vi "TLB Native Dynamic Events ver 0.15a.vi"() -> ()   [LabVIEW 2018]
uses:
  Labview Training Phase 2/Enum Controls/States for Action Engine.ctl
  TLB Type Definitions/State Type Definitions, for 0.26g versions and later 2.ctl
  TLB Type Definitions/Intruction Type Definitions.ctl
  TLB Type Definitions/Encoder cluster.ctl
  TLB Type Definitions/PING CLUSTER.ctl
  <vilib>/Studica/Studica Toolkit/NavX/NavX.lvlib
  <vilib>/Studica/Studica Toolkit/Background/DIO Channel.ctl
  Underlying VI's/NavX VI/navX type def.ctl
  <vilib>/myRIO/Instrument Drivers/Utilities/Utilities.lvlib
  <vilib>/Studica/Studica Toolkit/Background/I2C Channel.ctl
  TLB Type Definitions/Vision cluster.ctl
  <vilib>/NI_Real-Time Target Support.lvlib
  TLB Type Definitions/Stepper cluster.ctl
  Experimental VI's/Archived VI's/MOTOR CONTROL NO PID Type Def.ctl
  Underlying VI's/I2C Master VI/I2C MASTER Type Def.ctl
  Underlying VI's/I2C Master VI/I2C_MASTER_WRITE_NEW Type Def.ctl
  <vilib>/userdefined/High Color/IMAQdx.ctl
  Underlying VI's/I2C Master VI/Arduino_Interfacing.ctl
  TLB Type Definitions/Yaw Cluster.ctl
  Experimental VI's/Archived VI's/MOTOR CONTROL NO PID AE DATA ENTRY MODE Type def.ctl
  Experimental VI's/Archived VI's/MOTOR CONTROL NO PID AE DIRECTIONS type def.ctl
  Underlying VI's/Elasped Timer/Control.ctl
  TLB Type Definitions/Time cluster.ctl
  TLB Type Definitions/Y Stepper cluster.ctl
  Underlying VI's/Modified webcam FGV/Webcam AE.ctl
  <vilib>/Utility/RT CPU Load.ctl
panel:
  out "Does it leave this state?":bool
  out "Is object in range to pick up?":bool
  out "Does this get triged":bool
  out "Stepper position reached?":bool
  out "Cluster":T1
  out "Object Center Coordinates":cluster{"x":sgl, "y":sgl}
  out "Object detection cluster":T2
  out "Time up flag":bool
  out "Speed & distance":T3
  out "Task selection":u8
  in  "Object recognition mode":enum16{"Ball", "Soap", "Gel", "Pipe", "None"}(ring)
  out "NavX Readings":T4
  out "Arduino Data":T5
  out "CPU loads":T6[](array[typedef]) {"ISR (%)" format="%#.2f"; "Idle (%)" format="%#.2f"; "Background (%)" format="%#.2f"; "Normal (%)" format="%#.2f"; "Above Normal (%)" format="%#.2f"; "High (%)" format="%#.2g"; "Timed Structures (%)" format="%#.2g"; "Time Critical (%)" format="%#.2g"; "Total (%)" format="%#.2g"}
  out "TASK ENABLE":bool
  out "Rising Edge":bool
  in  "Green LED":bool
  out "Obstacle detected":bool
  out "I2C Error":errorcluster
  out "State Logic":T7=enum."Startup"
  out "elements":T8[](array[typedef])
  in  "STOP TASK":bool
  in  "OK Button":bool
  in  "STOP":bool
  out "error out":errorcluster
  out "Action Queue Items":i32
  out "State Logic Queue Items":i32
  out "Action Queues items":string[](array[string])=["Hardware reset", "Software reset", ""]
  out "Action State":string
  # "VISION"
  # "System Health Status Update"
  # "TLB FRAMEWORK STATUS"
  # "Test Programme written by Calvin Loke    Dated: 28 Aug 2019\nTest Programme revised by Dr Alex See   Dated 30 Aug 2019\n\nRevision date: 20/03/2020\nProgramme version:   TLB Native Dynamic Events ver 0.15a"
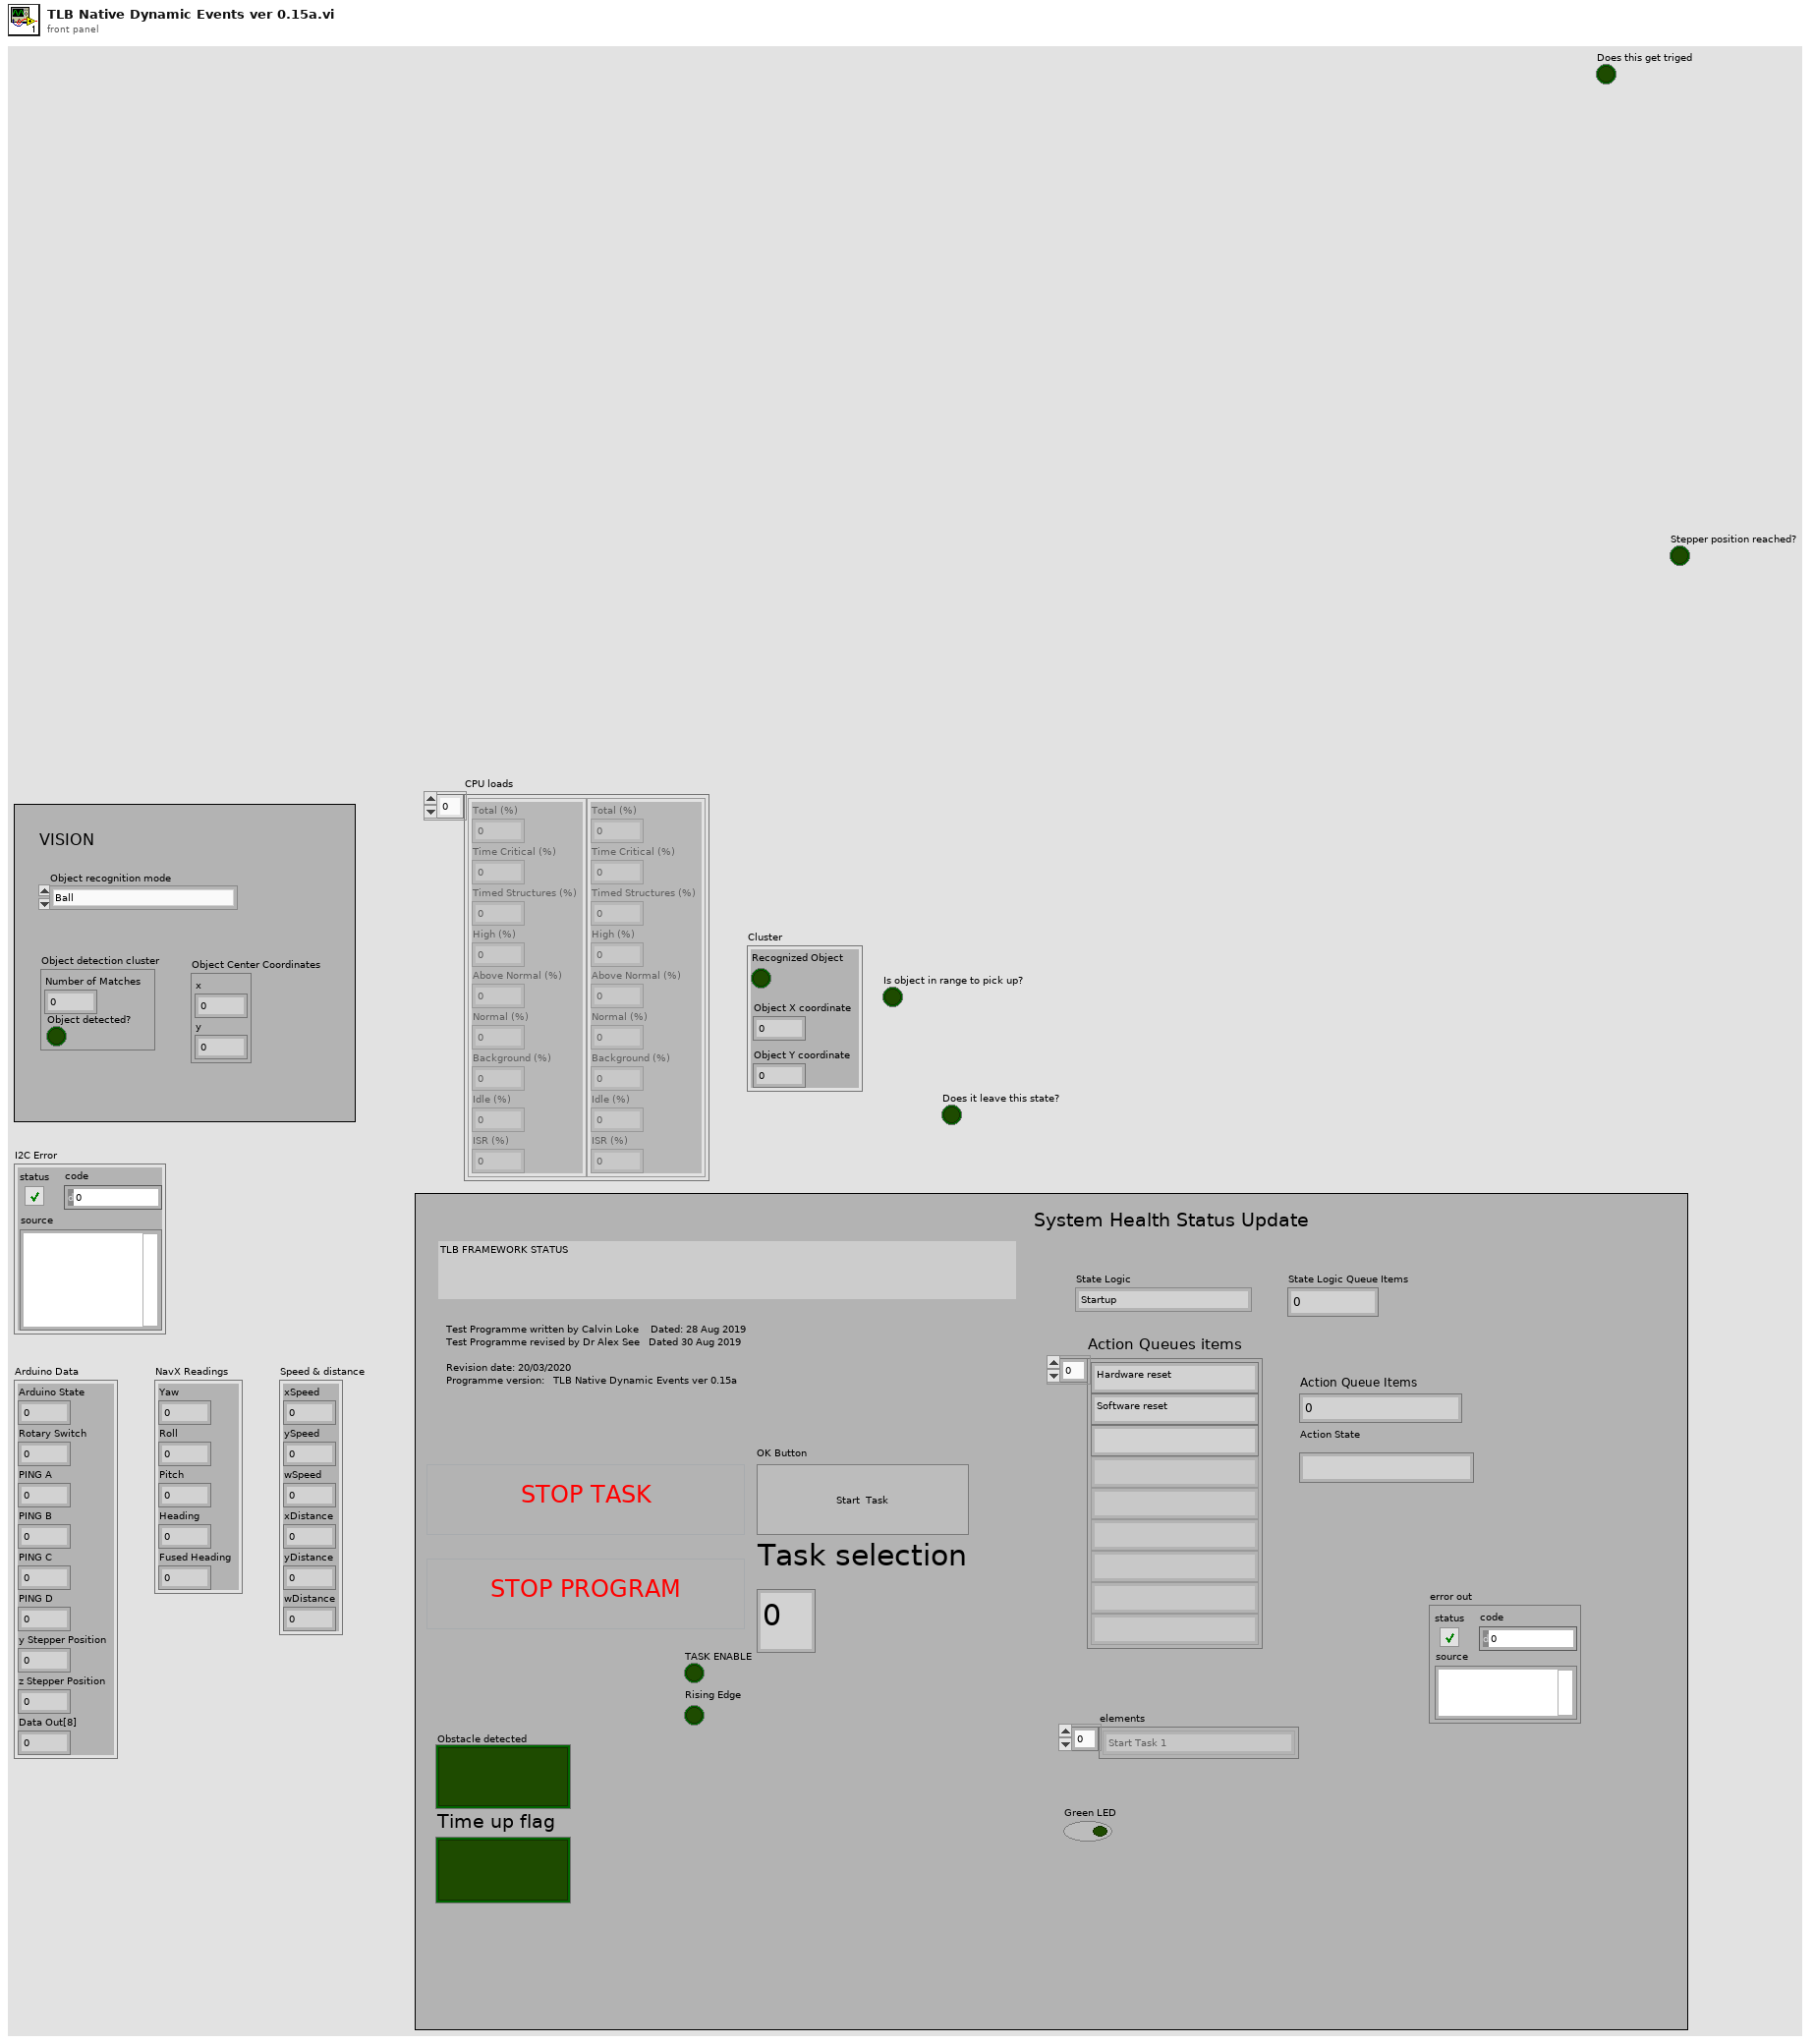
[diagram p1: front panel]
types:
  T1 = typedef "Vision cluster.ctl" = cluster{"Recognized Object":bool, "Object X coordinate":dbl, "Object Y coordinate":dbl}
  T2 = cluster{"Number of Matches":i32, "Object detected?":bool}
  T3 = cluster{"xSpeed":dbl, "ySpeed":dbl, "wSpeed":dbl, "xDistance":dbl, "yDistance":dbl, "wDistance":dbl}
  T4 = cluster{"Yaw":dbl, "Roll":dbl, "Pitch":dbl, "Heading":dbl, "Fused Heading":dbl}
  T5 = cluster{"Arduino State":u8, "Rotary Switch":u8, "PING A":u8, "PING B":u8, "PING C":u8, "PING D":u8, "y Stepper Position":u8, "z Stepper Position":u8, "Data Out[8]":u8}
  T6 = typedef "NI_Real-Time Target Support.lvlib/RT CPU Load.ctl" = cluster{"Total (%)":dbl, "Time Critical (%)":dbl, "Timed Structures (%)":dbl, "High (%)":dbl, "Above Normal (%)":dbl, "Normal (%)":dbl, "Background (%)":dbl, "Idle (%)":dbl, "ISR (%)":dbl}
  T7 = typedef "State Type Definitions, for 0.26g versions and later 2.ctl" = enum16{"None", "Startup", "Move to Angle", "True Stop", "Idle", "Shutdown", "Task 1A", "Task 1B", "Task 2:Raise Arm", "Task 2:Sensor Mode", "Task 2:Reverse Mode", "Task 3", "Task 4_A", "Task 4_B", "Task 4_C", "Task 4_D", "Task 5A", "Task 5B", "Task 5C", "Task 5D", "Task 5E: POSITION ARM", "Task 5F: ARM GRAB HEIGHT", "Task 5G: CLOSE CLAW", "Task 5H: RAISE ARM", "Task 6_A", "Task 6_B", "Task 7", "Task 8A: RAISE ARM", "Task 8B: MOVE TO BOX", "Task 8C: CAM BURST", "Task 8D: PROCESS IMAGE", "Task 8E: ROBOT ADJUST", "Task 8F: CAM BURST 2", "Task 8G: PROCESS IMAGE 2", "Task 8H: ARM ADJUST", "Task 8I: ARM GRAB HEIGHT", "Task 8J: CLOSE CLAW", "Task 8K: RAISE MY SWORD", "Task 9A: Raise Arm", "Task 9B: Rotate to Angle", "Task 9C: Detect Box", "Task 9D: MOVE FORWARD", "Task 9E: MOVE LEFT", "Task 9F: SCAN BOX", "Task 9G: MOVE RIGHT", "Task 9H: SCAN BOX 2", "Task 9I: ROTATE 90 CW", "Task 9J: FORWARD", "Task 9K: RAM WALL", "Task 9L: MOVE RIGHT", "Task 9M: SCAN BOX 3", "Task 9M: MOVE RIGHT", "Task 9N: SCAN BOX 4", "PENIS", "PENIS 2", "PENIS 3", "Task 9R: PROCESS COLOUR", "Task A1: Task 9 Open cam", "Task A2: Task 9 Move Arm", "Task A3: Task 9 Set Timer", "Task A4: Tasl 9 Capture images", "Task A5: Task 9 Close camera", "Task A6: Process Colour", "Task A7: Dispose Camera Buffer"}
  T8 = typedef "Intruction Type Definitions.ctl" = enum16{"None", "Start Task 1", "Start Task 2", "Start Task 3", "Start Task 4", "Start Task 5", "Start Task 6", "Start Task 7", "Start Task 8 - BALL", "Start Task 8 - Gel", "Start Task 8 - Pipe", "Start Task 8 - Soap", "Start Task 9", "Start Task A", "Start Task B", "Exit"}
  T9 = typedef "Y Stepper cluster.ctl" = cluster{"yStepper desired":u8}
  T10 = typedef "Time cluster.ctl" = cluster{"Time up flag":bool, "SET TIME TO CHECK":dbl}
  T11 = typedef "Yaw Cluster.ctl" = cluster{"Yaw":dbl, "Compass":dbl}
  T12 = typedef "Stepper cluster.ctl" = cluster{"y Stepper Position":u8, "z Stepper Position":u8}
  T13 = typedef "DIO Channel.ctl" = enum16{"Not Connected", "A/DIO1", "A/DIO2", "A/DIO3", "A/DIO4", "A/DIO5", "A/DIO6", "A/DIO7", "A/DIO13", "B/DIO1", "B/DIO2", "B/DIO3", "B/DIO4", "B/DIO5", "B/DIO6", "B/DIO7", "B/DIO13", "C/DIO0", "C/DIO1", "C/DIO2", "C/DIO3", "C/DIO4", "C/DIO5", "C/DIO6", "C/DIO7"}
  T14 = typedef "PING CLUSTER.ctl" = cluster{"PING_A":u8, "PING_B":u8, "PING_C":u8, "PING_D":u8}
  T15 = typedef "Encoder cluster.ctl" = cluster{"xDistance":dbl, "yDistance":dbl, "wDistance":dbl}
  T16 = cluster{"DIO Channel":T13, "FPGA VI Reference Out":refnum<k20>}
  T17 = typedef "MOTOR CONTROL NO PID AE DATA ENTRY MODE Type def.ctl" = enum16{"Initialize", "Reset Encoders", "Write to motors", "Read from Encoders"}
  T18 = typedef "navX type def.ctl" = enum16{"Get i2C reference", "Read Values", "Zero Yaw"}
  T19 = typedef "Arduino_Interfacing.ctl" = enum16{"Initialize", "Write to Arduino", "Read From Arduino"}
  T20 = typedef "I2C Channel.ctl" = enum16{"Not Connected", "A", "B"}
  T21 = typedef "States for Action Engine.ctl" = enum16{"Initialize", "Write", "Read"}
  T22 = cluster{"I2C Ref Out":cluster{"I2C Channel":T20, "FPGA VI Reference Out":refnum<k20>}, "Connected":bool, "Slave Address (7-bit)":u8, "Registry":u8[]}
  T23 = typedef "IMAQ Image.ctl" = refnum<image>
  T24 = typedef "State Type Definitions.ctl" = enum16{"None", "Startup", "Move to Angle", "True Stop", "Idle", "Shutdown", "Task 1", "Task 2", "Task 3", "Task 4_A", "Task 4_B", "Task 4_C", "Task 4_D", "Task 5_A", "Task 5 _B", "Task 5_C", "Task 5_D", "Task 5_D_Error", "Task 5D_Error_Right", "Task 5D_Error_Left", "Task 5_E", "Task 5_F", "Task 5F_Error", "Task 5G", "Task 5H", "Task 5I", "Task 6_A", "Task 6_B", "Task 7", "Task 8", "Task 9", "Task A", "Task B"}
  T25 = typedef "MOTOR CONTROL NO PID AE DIRECTIONS type def.ctl" = enum16{"y-axis movement", "x-axis movement", "Rotate", "Stop"}
  T26 = typedef "Control.ctl" = enum16{"Start", "Pause", "Initialize"}
  T27 = typedef "I2C_MASTER_WRITE_NEW Type Def.ctl" = enum16{"Ultrasonic sensors", "Stepper origin", "zStepper 13.3k", "zStepper 13k", "zStepper 12k", "zStepper 11k", "zStepper 10k", "zStepper 9k", "zStepper 8k", "zStepper 7k", "zStepper 6k", "zStepper 5k", "zStepper 4k", "zStepper 3k", "zStepper 2k", "zStepper 1k", "zStepper 900", "zStepper 800", "zStepper 700", "zStepper 600", "zStepper 500", "zStepper 400", "zStepper 300", "zStepper 200", "zStepper 100", "zStepper 0", "yStepper control", "Open Claw", "Close Claw", "Soft Reset"}
  T28 = typedef "Webcam AE.ctl" = enum16{"Initialize Camera", "Open Camera", "Continuous Acquisition", "Close Camera", "Retrieve Image", "Dispose Camera Image Buffer"}
  T29 = typedef "IMAQdx.ctl" = refnum<k21>
  T30 = typedef "Webcam AE.ctl" = enum16{"Initialize Camera", "Open Camera", "Continuous Acquisition", "Close Camera", "Retrieve Image", "Dispose Image Buffers"}
  T31 = typedef "MOTOR CONTROL NO PID Type Def.ctl" = enum16{"Init", "Front Back", "Left Right", "Rotate", "Stop", "Latch"}
  T32 = typedef "I2C MASTER Type Def.ctl" = enum16{"Last State", "Mode 0", "Mode 1", "Mode 2", "Mode 3", "Mode 4", "Mode 5", "Mode 6", "Mode 7", "Mode 8", "Mode 9", "Mode 10"}
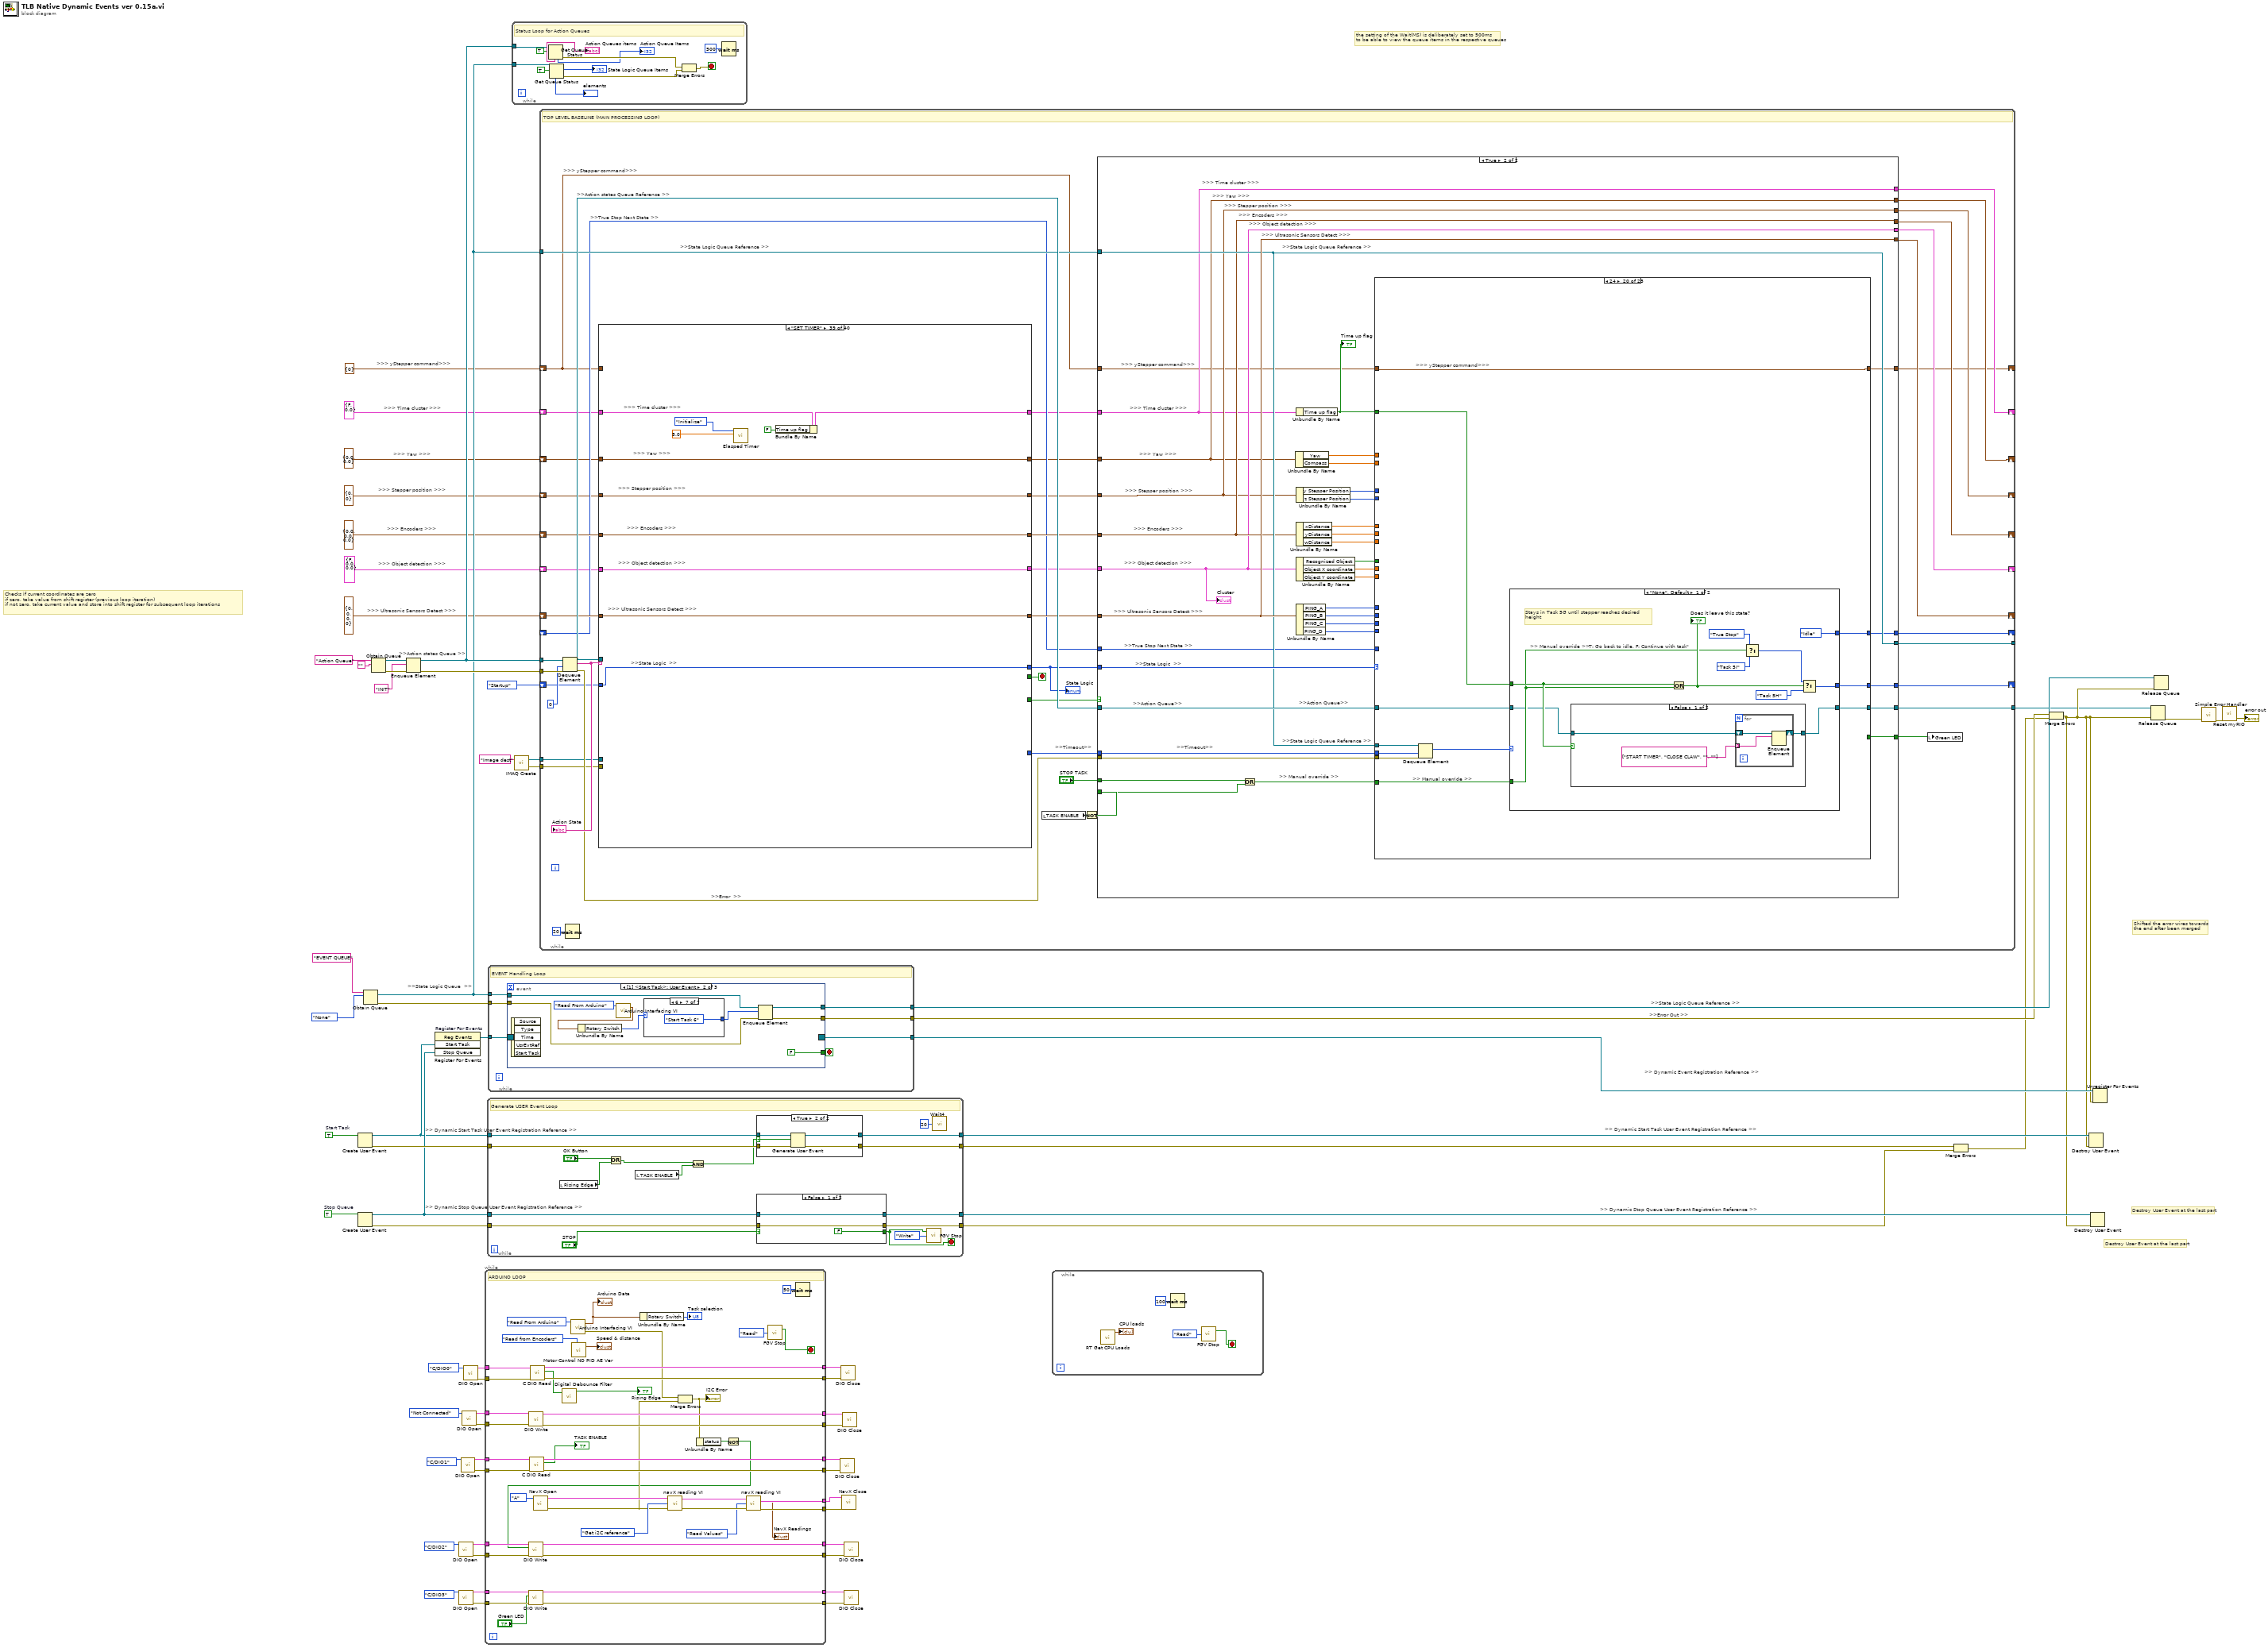
[diagram p0: block diagram]
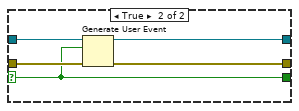
[diagram p2: hidden frame]
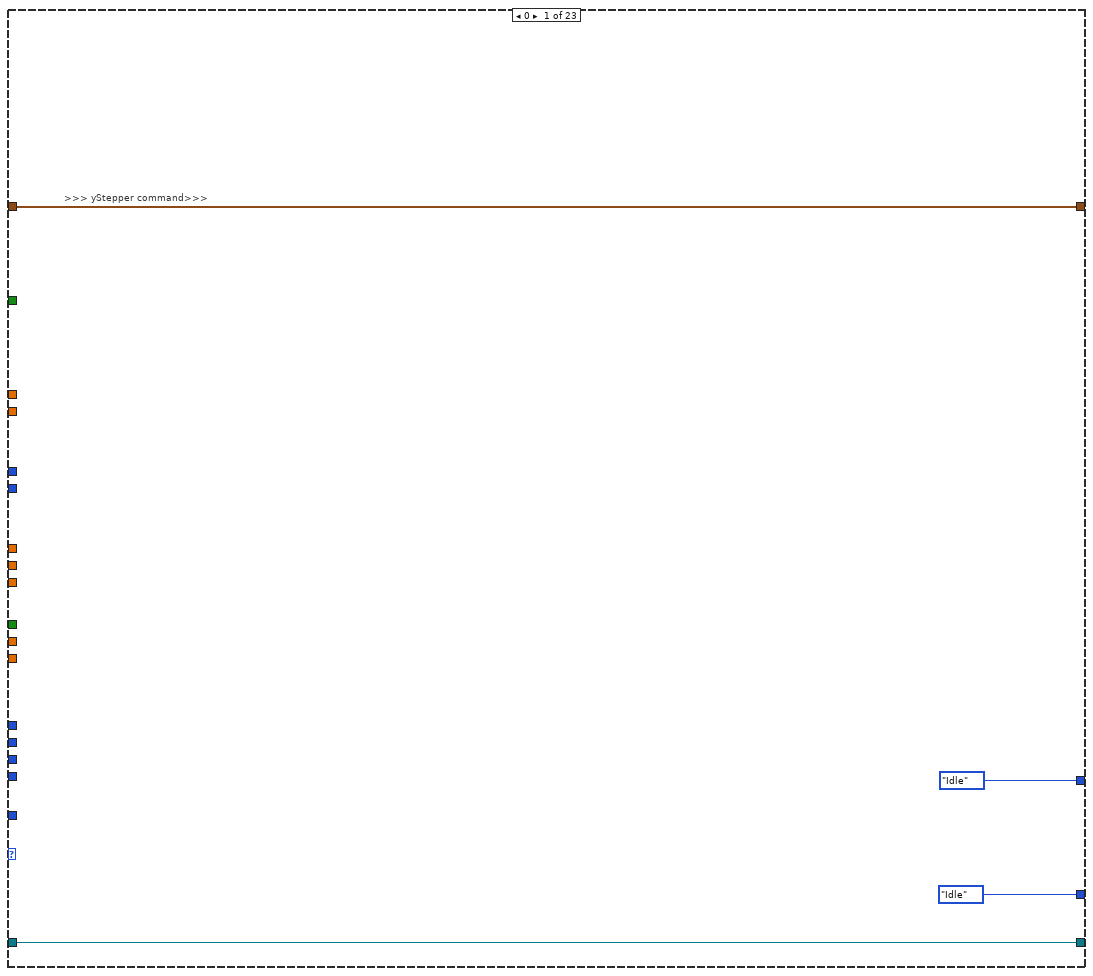
[diagram p5: hidden frame]
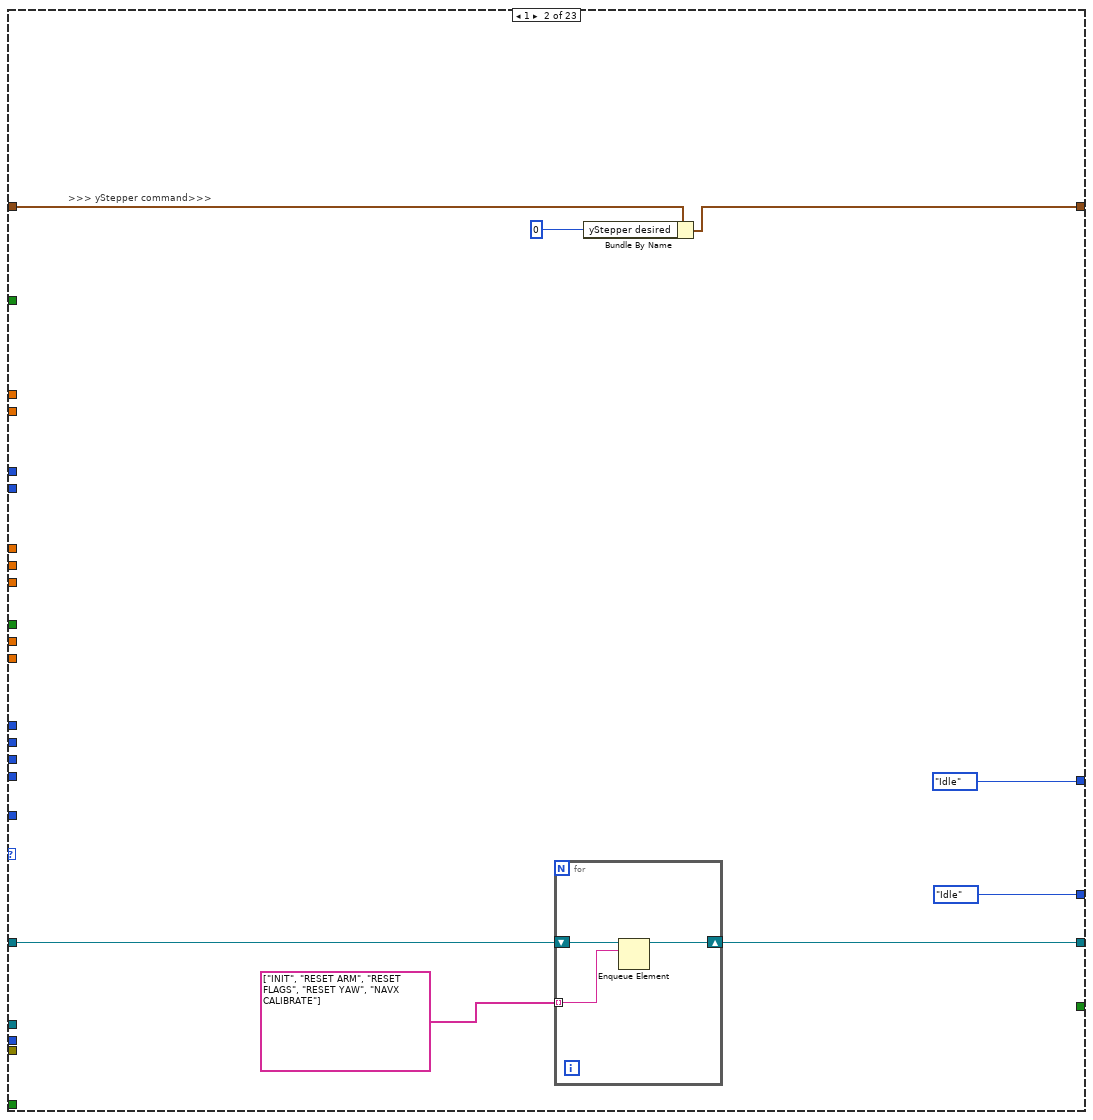
[diagram p6: hidden frame]
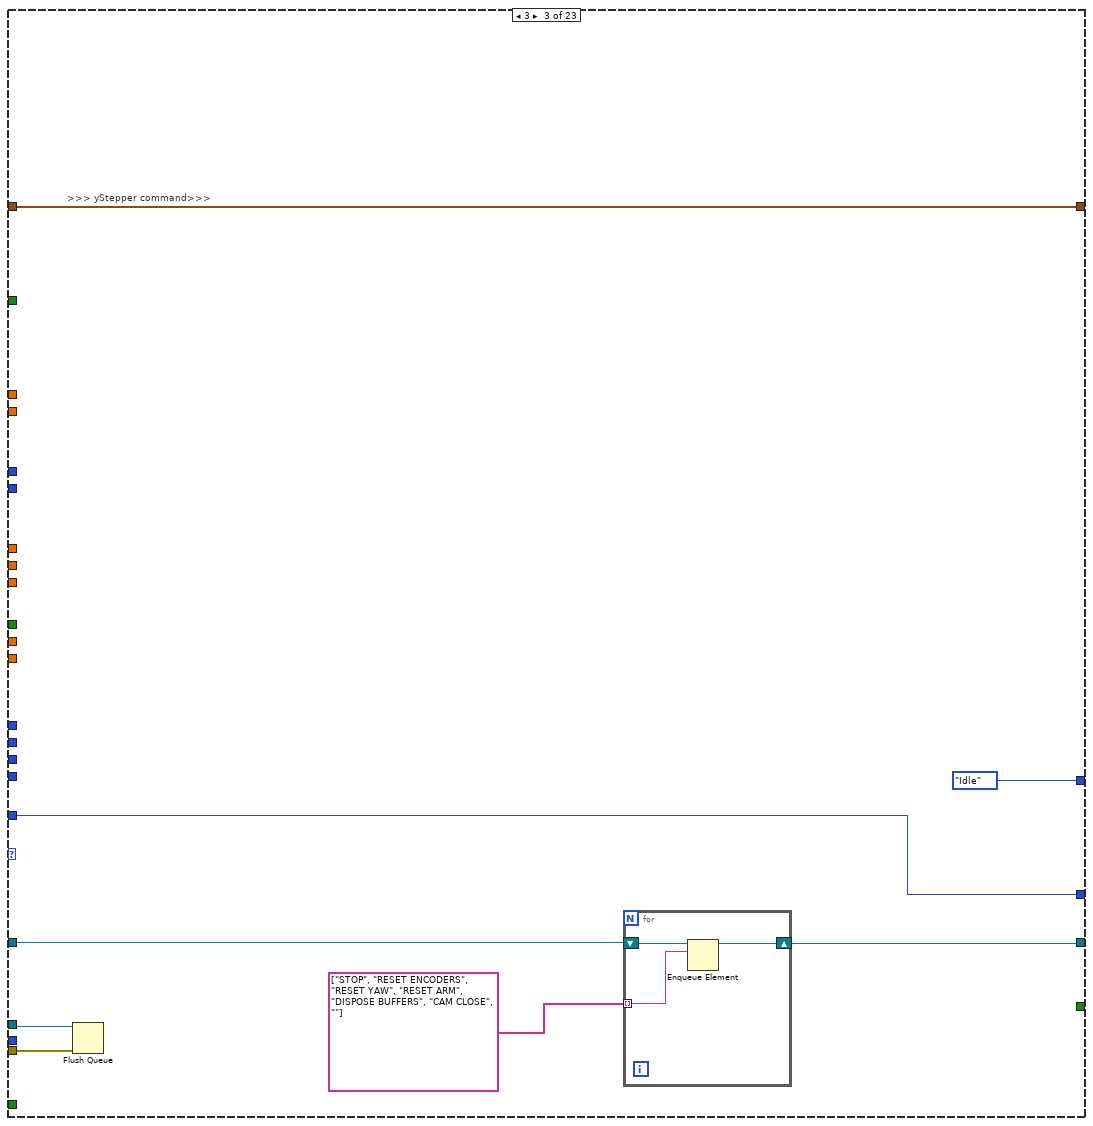
[diagram p7: hidden frame]
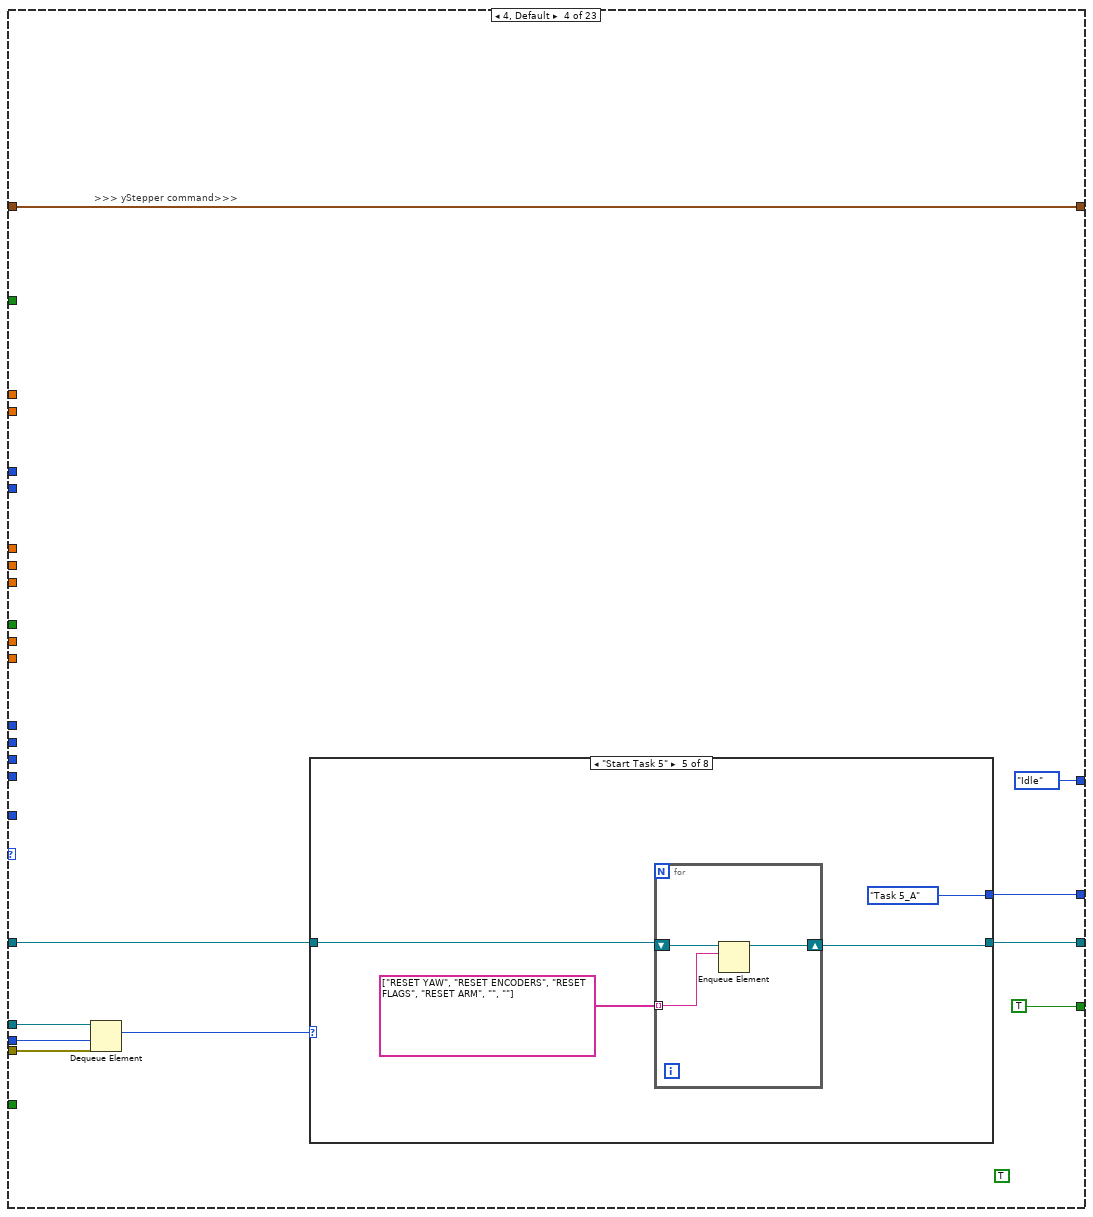
[diagram p8: hidden frame]
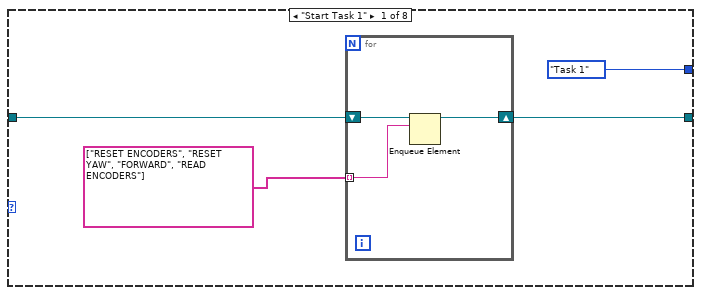
[diagram p9: hidden frame]
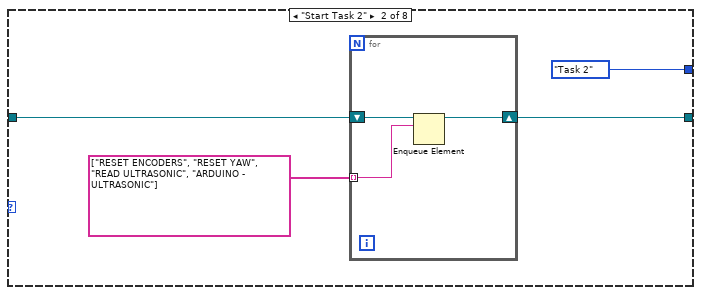
[diagram p10: hidden frame]
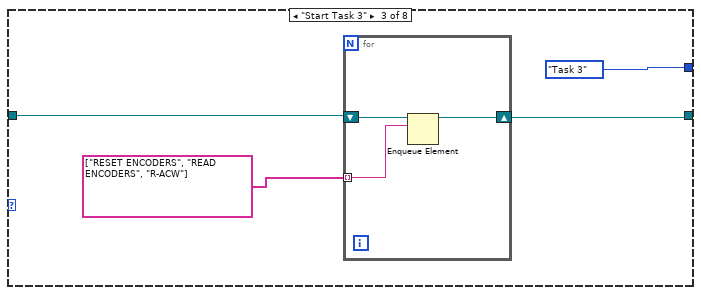
[diagram p11: hidden frame]
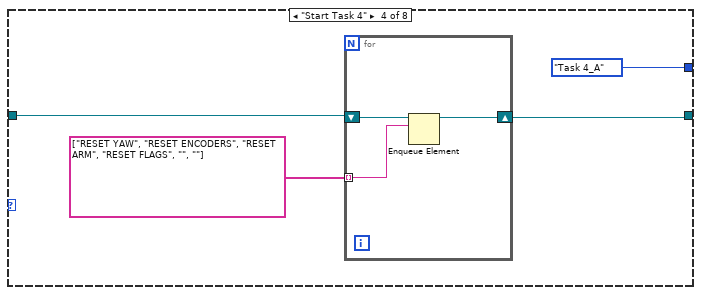
[diagram p12: hidden frame]
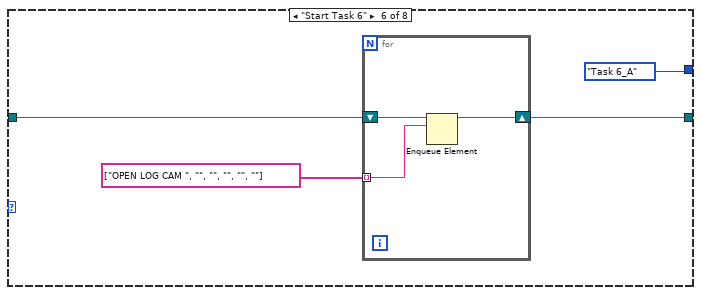
[diagram p13: hidden frame]
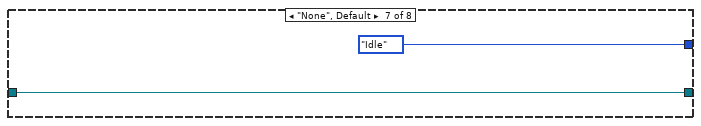
[diagram p14: hidden frame]
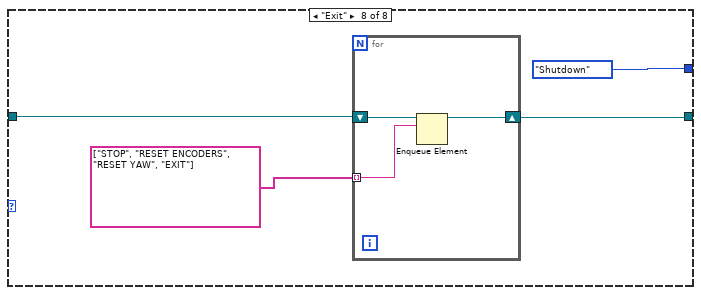
[diagram p15: hidden frame]
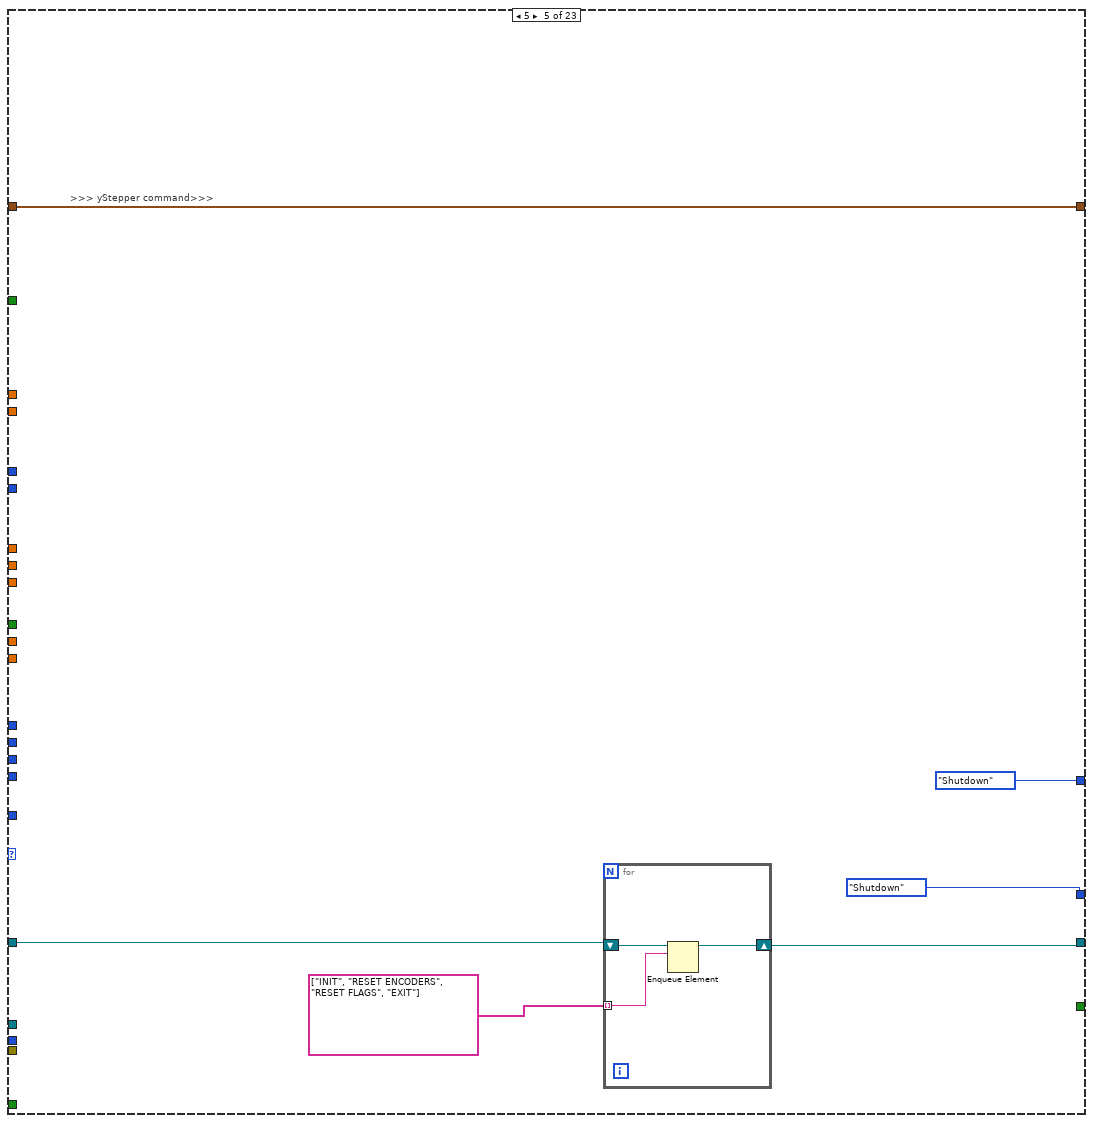
[diagram p16: hidden frame]
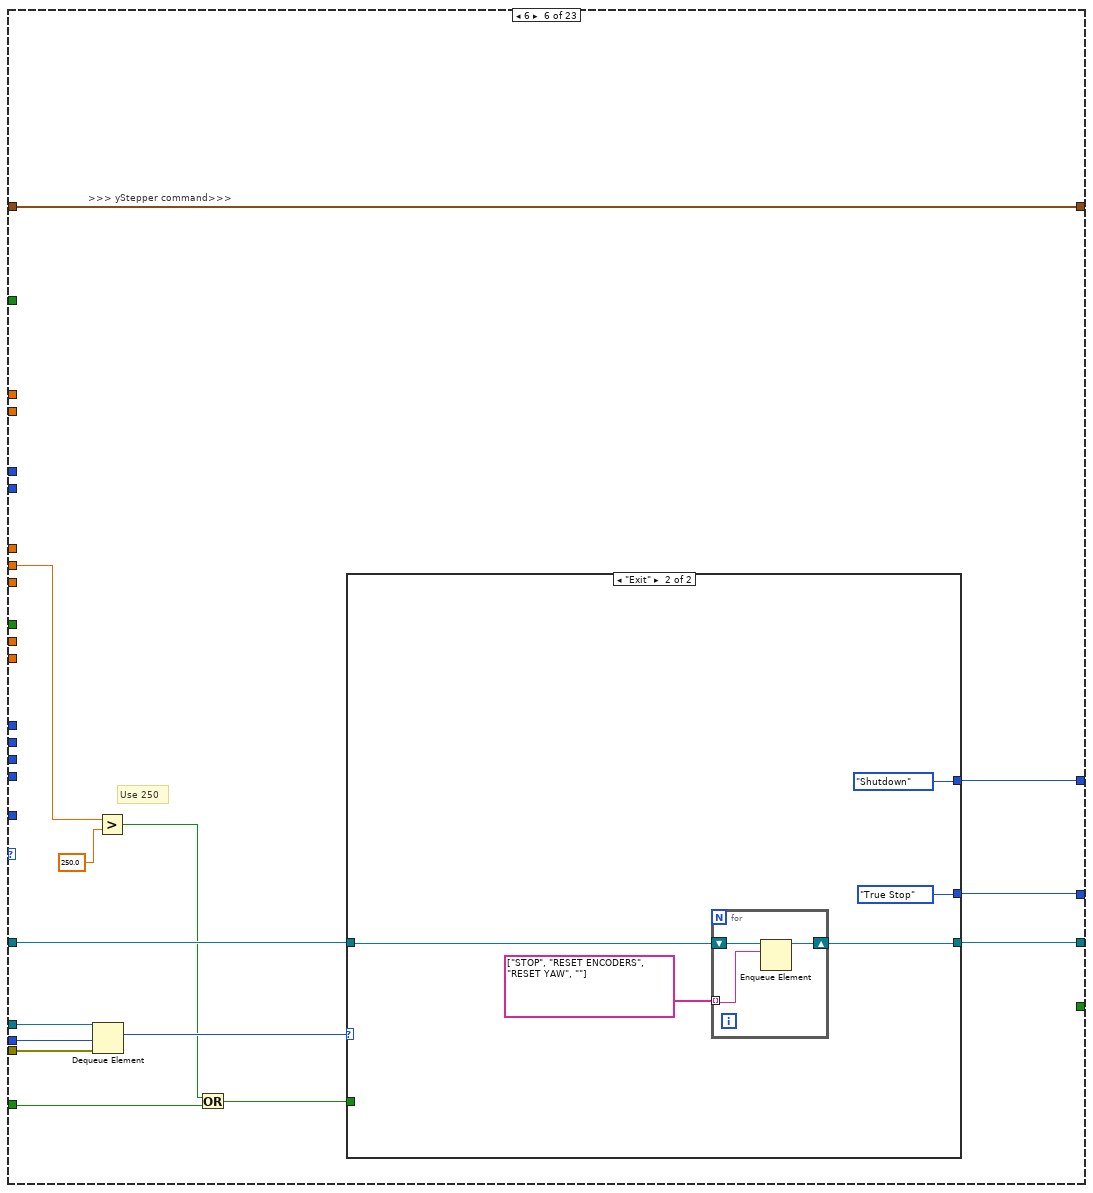
[diagram p17: hidden frame]
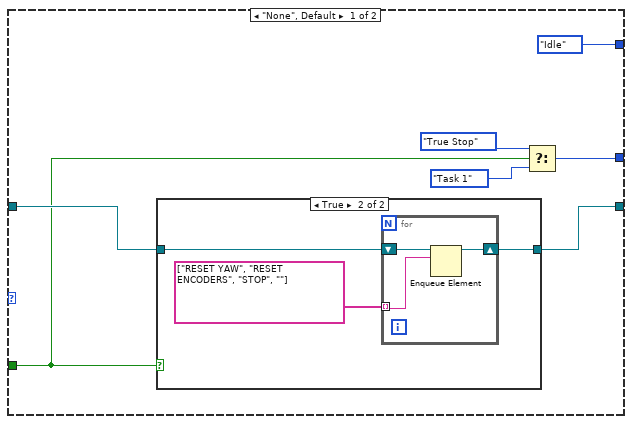
[diagram p18: hidden frame]
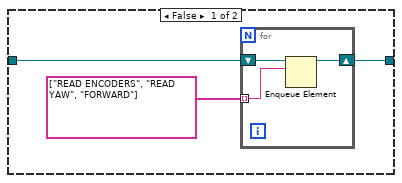
[diagram p19: hidden frame]
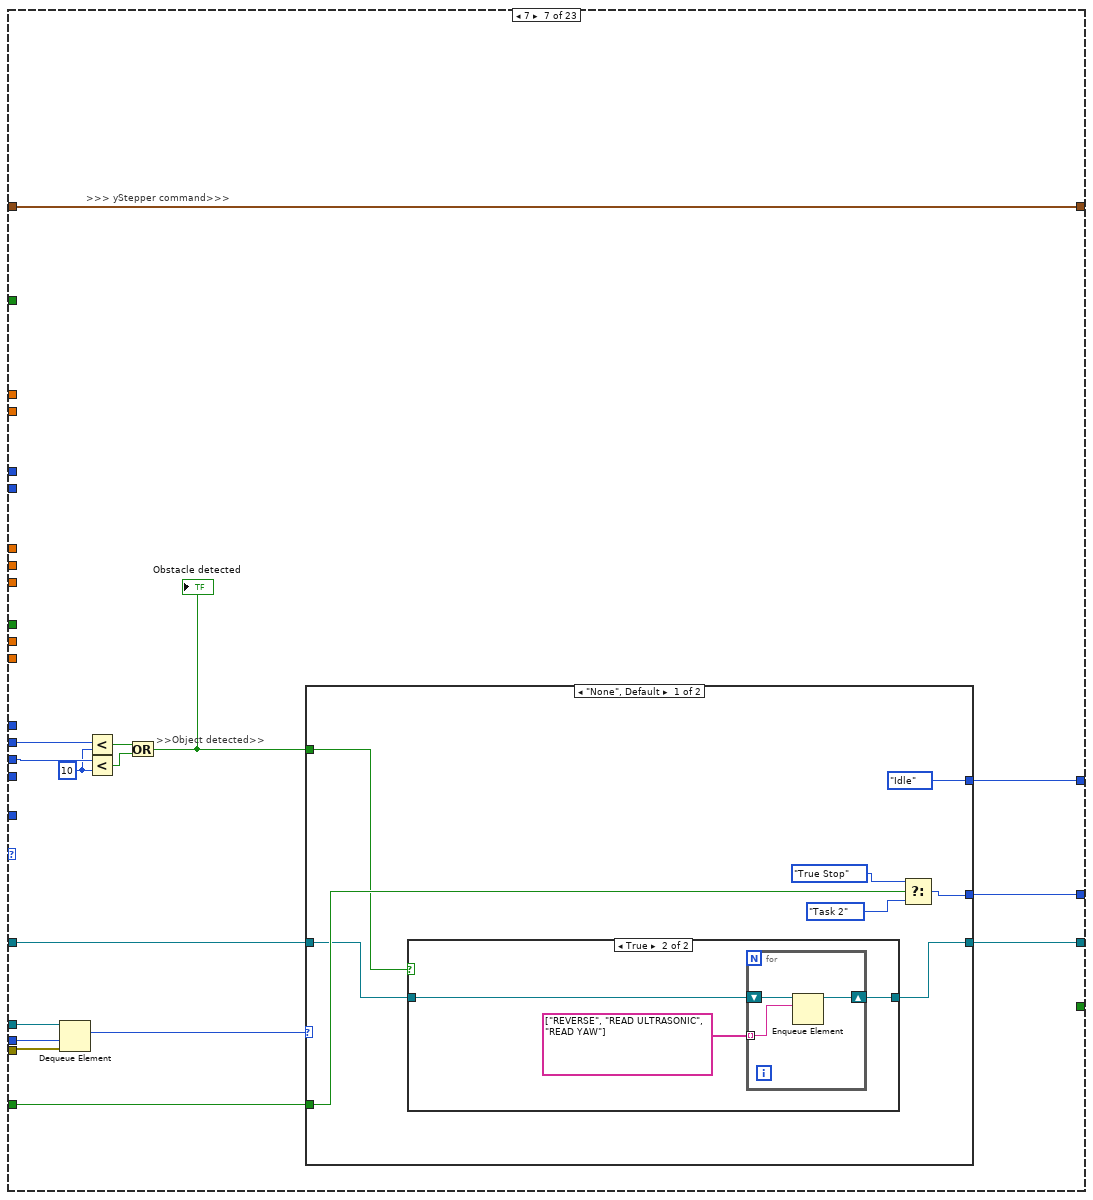
[diagram p20: hidden frame]
diagram:
  w69 = TRUE  # Stop Queue
  w68 = TRUE  # Start Task
  # "Checks if current coordinates are zero\nif zero, take value from shift register (previous loop iteration)\nif not zero, take current value and store into shift register for subsequent loop iterations"
  # ">>> yStepper command>>>"
  # ">>> Time cluster >>>"
  # ">>> Yaw >>>"
  # ">>> Stepper position >>>"
  # ">>> Encoders >>>"
  # ">>> Object detection >>>"
  # ">>> Ultrasonic Sensors Detect >>>"
  # "the setting of the Wait(MS) is deliberately set to 500ms\nto be able to view the queue items in the respective queues"
  # ">>Error Out >>"
  # ">> Dynamic Stop Queue User Event Registration Reference >>"
  # ">> Dynamic Start Task User Event Registration Reference >>"
  # ">> Dynamic Stop Queue User Event Registration Reference >>"
  # ">> Dynamic Start Task User Event Registration Reference >>"
  # ">> Dynamic Event Registration Reference >>"
  # ">>Action states Queue >>"
  # ">>State Logic Queue  >>"
  # ">>State Logic Queue Reference >>"
  # "Destroy User Event at the last part"
  # "Destroy User Event at the last part"
  # "Shifted the error wires towards\nthe end after been merged"
  n1 = Create User Event(user event datatype=w68) -> (user event=w60:refnum<user-event>, error out=w65:errorcluster)  [unwired: 1 in]
  n2 = Create User Event(user event datatype=w69) -> (user event=w61:refnum<user-event>, error out=w64:errorcluster)  [unwired: 1 in]
  n3 = Obtain Queue(name (unnamed)="EVENT QUEUE", element data type=Intruction_Type_Definitions."None" ("Enum")) -> (queue out=w46:refnum<queue>, error out=w52:errorcluster)  [unwired: 3 in, 1 out]
  n4 = Obtain Queue(name (unnamed)="Action Queue", element data type="") -> (queue out=w55:refnum<queue>, error out=w51:errorcluster)  [unwired: 3 in, 1 out]
  n5 = Enqueue Element(queue=w55, element="INIT", error in (no error)=w51) -> (queue out=w47:refnum<queue>, error out=w50:errorcluster)  [unwired: 1 in, 1 out]
  n6 = register-events "Register For Events"(w60, w61) -> (reference out=w59:refnum<event-registration>)  [unwired: 2 in, 1 out]
  n7 = call <vilib>:"DIO Open.vi"("DIO Channel"=DIO_Channel."C/DIO2") -> ("error out"=w14:errorcluster, "DIO Info Out"=w15:T16)  [unwired: 9 in]
  n8 = call <vilib>:"DIO Open.vi"("DIO Channel"=DIO_Channel."C/DIO3") -> ("error out"=w9:errorcluster, "DIO Info Out"=w10:T16)  [unwired: 9 in]
  n9 = call <vilib>:"DIO Open.vi"("DIO Channel"=DIO_Channel."C/DIO1") -> ("error out"=w25:errorcluster, "DIO Info Out"=w26:T16)  [unwired: 9 in]
  n10 = call <vilib>:"DIO Open.vi"("DIO Channel"=DIO_Channel."Not Connected") -> ("error out"=w30:errorcluster, "DIO Info Out"=w32:T16)  [unwired: 9 in]
  n11 = call <vilib>:"DIO Open.vi"("DIO Channel"=DIO_Channel."C/DIO0") -> ("error out"=w35:errorcluster, "DIO Info Out"=w38:T16)  [unwired: 9 in]
  n12 = while {
    tunnel: w38 -> [w112]
    tunnel: [w111] -> w36
    tunnel: w35 -> [w110]
    tunnel: [w109] -> w34
    tunnel: w32 -> [w106]
    tunnel: [w105] -> w31
    tunnel: w30 -> [w104]
    tunnel: [w103] -> w29
    tunnel: [w102] -> w27
    tunnel: w26 -> [w101]
    tunnel: w25 -> [w100]
    tunnel: [w99] -> w24
    tunnel: w15 -> [w93]
    tunnel: w14 -> [w92]
    tunnel: [w91] -> w13
    tunnel: [w90] -> w12
    tunnel: w10 -> [w89]
    tunnel: w9 -> [w88]
    tunnel: [w87] -> w8
    tunnel: [w86] -> w7
    tunnel: [w80] -> w4
    tunnel: [w79] -> w5
    stop <- w114 stop-if-true
    # "ARDUINO LOOP"
    n13 = call <vilib>:"DIO Write.vi"("error in (no error)"=w88, "Input"="Green LED", "DIO Info In"=w89) -> ("error out"=w86:errorcluster, "DIO Info Out"=w87:T16)  [unwired: 7 in]
    n14 = call <vilib>:"DIO Write.vi"("error in (no error)"=w104, "DIO Info In"=w106) -> ("error out"=w103:errorcluster, "DIO Info Out"=w105:T16)  [unwired: 8 in]
    n15 = call <vilib>:"C DIO Read.vi"("error in (no error)"=w100, "DIO Info In in"=w101) -> ("error out"=w99:errorcluster, "IN"=→"TASK ENABLE":bool, "DIO Info In out"=w102:T16)  [unwired: 7 in]
    n16 = call <vilib>:"C DIO Read.vi"("error in (no error)"=w110, "DIO Info In in"=w112) -> ("error out"=w109:errorcluster, "IN"=w108:bool, "DIO Info In out"=w111:T16)  [unwired: 7 in]
    n17 = call <vilib>:"NavX Open.vi"("I2C Channel"=I2C_Channel."A") -> ("error out"=w95:errorcluster, "NavX Info"=w97:T22)  [unwired: 9 in]
    n18 = call "Digital Debounce Filter.vi"("Boolean input"=w108) -> ("Rising Edge"=→"Rising Edge":bool)  [unwired: 1 in, 2 out]
    n19 = call "Arduino Interfacing VI.vi"("AE Mode"=Arduino_Interfacing."Read From Arduino") -> ("error out"=w83:errorcluster, "Arduino Data"=w76:T5)  [unwired: 3 in]
    "Arduino Data" <- w76
    n20 = call "Motor Control NO PID AE Ver.vi"("AE Mode"=MOTOR_CONTROL_NO_PID_AE_DATA_ENTRY_MODE_Type_def."Read from Encoders") -> ("Speed & distance"=→"Speed & distance":T3)  [unwired: 4 in, 1 out]
    n21 = Unbundle By Name(w76) -> ("Rotary Switch"=→"Task selection":u8)
    n22 = call "navX reading VI.vi"("NavX Info In"=w97, "Mode"=navX_type_def."Get i2C reference", "error in (no error)"=w95) -> ("NavX Info Out"=w82:T22, "Error Out"=w81:errorcluster)  [unwired: 2 out]
    n23 = Merge Errors(w83, w95) -> (w72:errorcluster)
    "I2C Error" <- w72
    n24 = Unbundle By Name(w72) -> ("status"=w71:bool)
    n25 = Not(x=w71) -> (.not. x?=w70:bool)
    n26 = call <vilib>:"DIO Write.vi"("error in (no error)"=w92, "Input"=w70, "DIO Info In"=w93) -> ("error out"=w90:errorcluster, "DIO Info Out"=w91:T16)  [unwired: 7 in]
    n27 = call "navX reading VI.vi"("NavX Info In"=w82, "Mode"=navX_type_def."Read Values", "error in (no error)"=w81) -> ("NavX Info Out"=w80:T22, "NavX Readings"=→"NavX Readings":T4, "Error Out"=w79:errorcluster)  [unwired: 1 out]
    n28 = call "FGV Stop.vi"("Init/Read/Write State"=States_for_Action_Engine."Read") -> ("Output node"=w114:bool)  [unwired: 2 in, 1 out]
    n29 = Wait (ms)(milliseconds to wait=u32 50) -> ()  [unwired: 1 out]
  }
  n30 = while {
    tunnel: w60 -> [w132]
    tunnel: w61 -> [w131]
    tunnel: [w130] -> w67
    tunnel: [w129] -> w66
    tunnel: w65 -> [w128]
    tunnel: [w127] -> w63
    tunnel: w64 -> [w126]
    tunnel: [w125] -> w62
    stop <- w123 stop-if-true
    # "Generate USER Event Loop"
    n31 = local read "Rising Edge"() -> (w119:bool)
    n32 = Or(x="OK Button", y=w119) -> (x .or. y?=w118:bool)
    n33 = local read "TASK ENABLE"() -> (w117:bool)
    n34 = And(x=w118, y=w117) -> (x .and. y?=w116:bool)
    n35 = case shown="True" w116 {
      selector: w116 -> [_ w143]
      tunnel: w132 -> [w142 w147]
      tunnel: [w142 w146] -> w129
      tunnel: w128 -> [w141 w145]
      tunnel: [w141 w144] -> w127
      frame False {
      }
      frame True {
        n36 = Generate User Event(user event=w147, event data cluster=w143, error in=w145) -> (user event out=w146:refnum<user-event>, error out=w144:errorcluster)  [unwired: 1 in]
      }
    }
    n37 = case shown="False" "STOP" {
      selector: "STOP" -> [_ w136]
      tunnel: w131 -> [w135 w140]
      tunnel: [w135 w139] -> w130
      tunnel: w126 -> [w134 w138]
      tunnel: [w134 w137] -> w125
      tunnel: [FALSE w136] -> w123
      frame False {
      }
      frame True {
        n38 = Generate User Event(user event=w140, event data cluster=w136, error in=w138) -> (user event out=w139:refnum<user-event>, error out=w137:errorcluster)  [unwired: 1 in]
      }
    }
    n39 = call "FGV Stop.vi"("Init/Read/Write State"=States_for_Action_Engine."Write", "Input Node"=w123) -> ()  [unwired: 1 in, 2 out]
    n40 = call "Wait4"("Count(uSec)"=u32 20) -> ()  [unwired: 1 out]
  }
  n41 = while {
    tunnel: w59 -> [w154]
    tunnel: [w153] -> w58
    tunnel: w46 -> [w151]
    tunnel: [w150] -> w57
    tunnel: w52 -> [w149]
    tunnel: [w148] -> w49
    stop <- w152 stop-if-true
    # "EVENT Handling Loop"
    n42 = event shown="[1] <Start Task>: User Event" {
      selector: w154 -> [_ _ _]
      dyn-events: [_ _ _] -> w153
      timeout: _ -> [_ _ _]
      tunnel: [FALSE FALSE w182] -> w152
      tunnel: w151 -> [w159 w168 w180]
      tunnel: [w158 w167 w181] -> w150
      tunnel: w149 -> [w157 w166 w179]
      tunnel: [w156 w165 w178] -> w148
      event Timeout {
        n43 = event-data() -> ()  [unwired: 1 in, 3 out]
        n44 = Enqueue Element(queue=w159, element=Intruction_Type_Definitions."None" ("Enum"), error in (no error)=w157) -> (queue out=w158:refnum<queue>, error out=w156:errorcluster)  [unwired: 1 in, 1 out]
      }
      event User Event {
        n45 = event-data() -> ()  [unwired: 1 in, 5 out]
        n46 = call "Arduino Interfacing VI.vi"("AE Mode"=Arduino_Interfacing."Read From Arduino") -> ("Arduino Data"=w162:T5)  [unwired: 3 in, 1 out]
        n47 = Unbundle By Name(w162) -> ("Rotary Switch"=w161:u8)
        n48 = case shown="6" w161 {
          tunnel: [Intruction_Type_Definitions."None" ("Enum") Intruction_Type_Definitions."Start Task 1" ("Enum") Intruction_Type_Definitions."Start Task 2" ("Enum") Intruction_Type_Definitions."Start Task 3" ("Enum") Intruction_Type_Definitions."Start Task 4" ("Enum") Intruction_Type_Definitions."Start Task 5" ("Enum") Intruction_Type_Definitions."Start Task 6" ("Enum")] -> w164
          frame 0, Default {
          }
          frame 1 {
          }
          frame 2 {
          }
          frame 3 {
          }
          frame 4 {
          }
          frame 5 {
          }
          frame 6 {
          }
        }
        n49 = Enqueue Element(queue=w168, element=w164, error in (no error)=w166) -> (queue out=w167:refnum<queue>, error out=w165:errorcluster)  [unwired: 1 in, 1 out]
      }
      event User Event {
        n50 = event-data() -> ("Stop Queue"=w182:bool)  [unwired: 1 in, 4 out]
        n51 = Enqueue Element At Opposite End(queue=w180, element=Intruction_Type_Definitions."Exit" ("Enum"), error in (no error)=w179) -> (queue out=w181:refnum<queue>, error out=w178:errorcluster)  [unwired: 1 in, 1 out]
      }
    }
  }
  n52 = while {
    tunnel: w47 -> [w192]
    tunnel: w46 -> [w189]
    stop <- w186 stop-if-true
    # "Status Loop for Action Queues"
    n53 = Get Queue Status(queue=w192, return elements? (F)=TRUE) -> (error out=w188:errorcluster, # elements in queue=→"Action Queue Items":i32, elements=→"Action Queues items":string[])  [unwired: 1 in, 5 out]
    n54 = Get Queue Status(queue=w189, return elements? (F)=TRUE) -> (# pending remove=→"State Logic Queue Items":i32, error out=w187:errorcluster, elements=→"elements":T8[])  [unwired: 1 in, 5 out]
    n55 = Merge Errors(w188, w187) -> (w186:errorcluster)
    n56 = Wait (ms)(milliseconds to wait=u32 500) -> ()  [unwired: 1 out]
  }
  n57 = call "IMAQ Create"("Image Name"="Image dest") -> ("New Image"=w19:T23, "error out"=w18:errorcluster)  [unwired: 4 in]
  n58 = while {
    tunnel: w46 -> [w226]
    tunnel: w47 -> [w238]
    tunnel: w50 -> [w236]
    tunnel: [w235] -> _
    tunnel: [w234] -> w40
    shift-right: [w227] -> _
    shift-left: T14 {"PING_A"=0, "PING_B"=0, "PING_C"=0, "PING_D"=0} -> [w229]
    shift-right: [w220] -> _
    shift-left: State_Type_Definitions,_for_0.26g_versions_and_later_2."Startup" ("Enum") -> [w223]
    shift-right: [w216] -> _
    shift-left: T15 {"xDistance"=0.0, "yDistance"=0.0, "wDistance"=0.0} -> [w218]
    shift-right: [w213] -> _
    shift-left: _ -> [w212]
    tunnel: w19 -> [w211]
    tunnel: w18 -> [w210]
    shift-right: [w207] -> _
    shift-left: T1 {"Recognized Object"=FALSE, "Object X coordinate"=0.0, "Object Y coordinate"=0.0} -> [w209]
    shift-right: [w204] -> _
    shift-left: T12 {"y Stepper Position"=0, "z Stepper Position"=0} -> [w206]
    shift-right: [w201] -> _
    shift-left: T11 {"Yaw"=0.0, "Compass"=0.0} -> [w203]
    shift-right: [w198] -> _
    shift-left: T10 {"Time up flag"=FALSE, "SET TIME TO CHECK"=0.0} -> [w200]
    shift-right: [w196] -> _
    shift-left: T9 {"yStepper desired"=0} -> [w197]
    stop <- w225 stop-if-true
    # ">>> yStepper command>>>"
    # ">>True Stop Next State >>"
    # ">>Error  >>"
    # ">>Timeout>>"
    # ">>Action states Queue Reference >>"
    # ">>State Logic Queue Reference >>"
    # "TOP LEVEL BASELINE (MAIN PROCESSING LOOP)"
    n59 = Dequeue Element(queue=w238, timeout in ms (-1)=0, error in (no error)=w236) -> (queue out=w230:refnum<queue>, element=w237:string, error out=w231:errorcluster)  [unwired: 1 out]
    "Action State" <- w237
    n60 = Wait (ms)(milliseconds to wait=u32 20) -> ()  [unwired: 1 out]
    n61 = case shown="\"SET TIMER\"" w237 {
      tunnel: [_ _ _ _ _ _ _ _ _ _ _ _ _ _ _ _ 0 w1350 _ _ _ _ _ _ _ _ _ _ _ _ _ _ _ _ _ _ _ _ _ _] -> w233
      tunnel: w230 -> [_ _ _ _ _ _ _ _ _ _ _ _ _ _ _ _ _ _ _ _ _ _ _ _ _ _ _ _ _ _ _ _ _ _ _ _ _ _ _ _]
      tunnel: w229 -> [w1165 w1173 w1184 w1195 w1205 w1215 w1226 w1237 w1247 w1253 w1267 w1280 w1291 w1299 w1323 w1332 w1342 w1351 w1359 w1367 w1396 w1406 w1413 w1421 w1433 w1445 w1454 w1462 w1478 w1486 w1496 w1505 w1514 w1523 w1529 w1540 w1555 w1560 w1571 w1581]
      tunnel: [w1165 w1173 w1184 w1195 w1205 w1215 w1226 w1237 w1247 w1253 w1267 w1281 w1291 w1299 w1324 w1332 w1342 w1351 w1359 w1367 w1395 w1406 w1413 w1421 w1433 w1445 w1454 w1462 w1478 w1486 w1496 w1505 w1514 w1523 w1529 w1540 w1555 w1560 w1571 w1581] -> w228
      tunnel: [TRUE TRUE _ _ _ _ _ _ _ _ _ _ _ _ _ _ _ _ _ _ _ _ _ _ _ _ _ _ _ _ _ _ _ _ _ _ _ _ _ _] -> w225
      tunnel: w223 -> [w1163 w1171 w1183 w1194 w1204 w1214 w1225 w1236 w1246 w1252 w1266 w1279 w1290 w1298 w1322 w1331 w1339 w1348 w1358 w1366 w1394 w1405 w1412 w1420 w1432 w1444 w1453 w1461 w1477 w1485 w1495 w1504 w1513 w1522 w1528 w1539 w1554 w1559 w1570 w1580]
      tunnel: [_ _ _ _ _ _ _ _ _ _ _ _ _ _ _ _ _ TRUE _ _ _ _ _ _ _ _ _ _ _ _ _ _ _ _ _ _ _ _ _ _] -> w222
      tunnel: [w1163 w1171 w1183 w1194 w1204 w1214 w1225 w1236 w1246 w1252 w1266 w1279 w1290 w1298 w1322 w1331 w1339 w1348 w1358 w1366 w1394 w1405 w1412 w1420 w1432 w1444 w1453 w1461 w1477 w1485 w1495 w1504 w1513 w1522 w1528 w1539 w1554 w1559 w1570 w1580] -> w221
      tunnel: w218 -> [w1162 w1170 w1182 w1193 w1203 w1213 w1224 w1235 w1245 w1254 w1265 w1278 w1292 w1300 w1321 w1333 w1338 w1347 w1360 w1368 w1384 w1404 w1415 w1422 w1434 w1446 w1455 w1463 w1479 w1488 w1498 w1507 w1516 w1525 w1531 w1542 w1557 w1562 w1573 w1583]
      tunnel: [w1162 w1170 w1182 w1193 w1203 w1213 w1224 w1235 w1245 w1254 w1264 w1278 w1292 w1300 w1320 w1333 w1338 w1347 w1360 w1368 w1383 w1404 w1415 w1422 w1434 w1446 w1455 w1463 w1479 w1488 w1498 w1507 w1516 w1525 w1531 w1542 w1557 w1562 w1573 w1583] -> w217
      tunnel: w211 -> [w1157 _ _ _ _ _ _ _ _ _ _ _ _ _ _ _ _ _ _ _ _ _ _ _ _ _ _ _ w1473 _ _ _ _ _ _ _ _ _ _ _]
      tunnel: w210 -> [_ _ _ _ _ _ _ _ _ _ _ _ _ _ _ _ _ _ _ _ _ _ _ _ _ _ w1447 _ w1475 w1484 _ _ _ _ _ _ _ _ _ _]
      tunnel: w209 -> [w1161 w1169 w1181 w1192 w1202 w1212 w1223 w1234 w1243 w1251 w1263 w1277 w1285 w1297 w1312 w1330 w1337 w1346 w1357 w1365 w1389 w1402 w1414 w1419 w1431 w1443 w1449 w1460 w1470 w1487 w1497 w1506 w1515 w1524 w1530 w1541 w1556 w1561 w1572 w1582]
      tunnel: [w1161 w1169 w1181 w1192 w1202 w1212 w1223 w1234 w1243 w1251 w1263 w1277 w1285 w1297 w1311 w1330 w1337 w1346 w1357 w1365 w1388 w1402 w1414 w1419 w1431 w1443 w1449 w1460 w1469 w1487 w1497 w1506 w1515 w1524 w1530 w1541 w1556 w1561 w1572 w1582] -> w208
      tunnel: w206 -> [w1160 w1168 w1180 w1191 w1201 w1211 w1222 w1233 w1242 w1250 w1262 w1276 w1293 w1296 w1317 w1329 w1336 w1345 w1356 w1364 w1379 w1401 w1411 w1418 w1430 w1442 w1452 w1459 w1480 w1489 w1494 w1503 w1512 w1521 w1532 w1543 w1553 w1563 w1574 w1584]
      tunnel: [w1160 w1168 w1180 w1191 w1201 w1211 w1222 w1233 w1242 w1250 w1262 w1276 w1293 w1296 w1316 w1329 w1336 w1345 w1356 w1364 w1378 w1401 w1411 w1418 w1430 w1442 w1452 w1459 w1480 w1489 w1494 w1503 w1512 w1521 w1532 w1543 w1552 w1563 w1574 w1584] -> w205
      tunnel: w203 -> [w1159 w1167 w1175 w1186 w1196 w1210 w1217 w1228 w1241 w1249 w1256 w1269 w1288 w1295 w1307 w1328 w1335 w1344 w1355 w1363 w1375 w1400 w1408 w1417 w1429 w1441 w1451 w1458 w1481 w1490 w1493 w1500 w1509 w1518 w1533 w1544 w1547 w1564 w1575 w1585]
      tunnel: [w1159 w1167 w1175 w1186 w1196 w1210 w1217 w1228 w1241 w1249 w1256 w1269 w1287 w1295 w1306 w1328 w1335 w1344 w1355 w1363 w1374 w1400 w1408 w1417 w1429 w1441 w1451 w1458 w1481 w1490 w1493 w1500 w1509 w1518 w1533 w1544 w1547 w1564 w1575 w1585] -> w202
      tunnel: w200 -> [w1156 w1166 w1176 w1187 w1197 w1206 w1218 w1229 w1238 w1248 w1255 w1268 w1284 w1294 w1301 w1325 w1334 w1343 w1354 w1361 w1372 w1398 w1407 w1416 w1428 w1440 w1450 w1457 w1482 w1491 w1492 w1499 w1508 w1517 w1534 w1545 w1546 w1558 w1568 w1578]
      tunnel: [w1156 w1166 w1176 w1187 w1197 w1206 w1218 w1229 w1238 w1248 w1255 w1268 w1284 w1294 w1301 w1325 w1334 w1343 w1354 w1361 w1371 w1398 w1407 w1416 w1428 w1440 w1450 w1457 w1482 w1491 w1492 w1499 w1508 w1517 w1534 w1545 w1546 w1558 w1566 w1577] -> w199
      tunnel: w197 -> [_ _ _ _ _ _ _ _ _ _ _ _ _ _ _ _ _ _ _ _ _ _ _ _ _ _ _ _ _ _ _ _ _ _ _ w1536 _ _ _ _]
      frame "Exit" {
        # ">>State Logic  >>"
        # ">>> Time cluster >>>"
        # ">>> Yaw >>>"
        # ">>> Stepper position >>>"
        # ">>> Encoders >>>"
        # ">>> Object detection >>>"
        # ">>> Ultrasonic Sensors Detect >>>"
        n62 = call "Imaq Dispose"("All Images? (No)"=TRUE, "Image"=w1157) -> ()  [unwired: 4 in, 1 out]
      }
      frame "----Movement States----" {
        # ">>State Logic  >>"
        # ">>> Time cluster >>>"
        # ">>> Yaw >>>"
        # ">>> Stepper position >>>"
        # ">>> Encoders >>>"
        # ">>> Object detection >>>"
        # ">>> Ultrasonic Sensors Detect >>>"
      }
      frame "FORWARD" {
        # ">>> Time cluster >>>"
        # ">>> Yaw >>>"
        # ">>> Stepper position >>>"
        # ">>> Encoders >>>"
        # ">>> Object detection >>>"
        # ">>> Ultrasonic Sensors Detect >>>"
        n63 = Unbundle By Name(w1175) -> ("Yaw"=w1174:dbl)
        n64 = call "Motor Control NO PID AE Ver.vi"("Direction"=MOTOR_CONTROL_NO_PID_AE_DIRECTIONS_type_def."y-axis movement", "AE Mode"=MOTOR_CONTROL_NO_PID_AE_DATA_ENTRY_MODE_Type_def."Write to motors", "Speed"=0.5, "Yaw"=w1174) -> ()  [unwired: 1 in, 2 out]
      }
      frame "LEFT" {
        # ">>State Logic  >>"
        # ">>> Time cluster >>>"
        # ">>> Yaw >>>"
        # ">>> Stepper position >>>"
        # ">>> Encoders >>>"
        # ">>> Object detection >>>"
        # ">>> Ultrasonic Sensors Detect >>>"
        n65 = Unbundle By Name(w1186) -> ("Yaw"=w1185:dbl)
        n66 = call "Motor Control NO PID AE Ver.vi"("Direction"=MOTOR_CONTROL_NO_PID_AE_DIRECTIONS_type_def."x-axis movement", "AE Mode"=MOTOR_CONTROL_NO_PID_AE_DATA_ENTRY_MODE_Type_def."Write to motors", "Speed"=-0.5, "Yaw"=w1185) -> ()  [unwired: 1 in, 2 out]
      }
      frame "R-ACW" {
        n67 = call "Motor Control NO PID AE Ver.vi"("Direction"=MOTOR_CONTROL_NO_PID_AE_DIRECTIONS_type_def."Rotate", "AE Mode"=MOTOR_CONTROL_NO_PID_AE_DATA_ENTRY_MODE_Type_def."Write to motors", "Speed"=0.25) -> ()  [unwired: 2 in, 2 out]
      }
      frame "R-CW" {
        (unwired) -0.2 ("Speed")
        n68 = call "Motor Control NO PID AE Ver.vi"("Direction"=MOTOR_CONTROL_NO_PID_AE_DIRECTIONS_type_def."Rotate", "AE Mode"=MOTOR_CONTROL_NO_PID_AE_DATA_ENTRY_MODE_Type_def."Write to motors", "Speed"=-0.5) -> ()  [unwired: 2 in, 2 out]
      }
      frame "RIGHT" {
        n69 = Unbundle By Name(w1217) -> ("Yaw"=w1216:dbl)
        n70 = call "Motor Control NO PID AE Ver.vi"("Direction"=MOTOR_CONTROL_NO_PID_AE_DIRECTIONS_type_def."x-axis movement", "AE Mode"=MOTOR_CONTROL_NO_PID_AE_DATA_ENTRY_MODE_Type_def."Write to motors", "Speed"=0.5, "Yaw"=w1216) -> ()  [unwired: 1 in, 2 out]
      }
      frame "REVERSE" {
        n71 = Unbundle By Name(w1228) -> ("Yaw"=w1227:dbl)
        n72 = call "Motor Control NO PID AE Ver.vi"("Direction"=MOTOR_CONTROL_NO_PID_AE_DIRECTIONS_type_def."y-axis movement", "AE Mode"=MOTOR_CONTROL_NO_PID_AE_DATA_ENTRY_MODE_Type_def."Write to motors", "Speed"=-0.5, "Yaw"=w1227) -> ()  [unwired: 1 in, 2 out]
      }
      frame "STOP" {
        n73 = Wait (ms)(milliseconds to wait=u32 500) -> ()  [unwired: 1 out]
        n74 = call "Motor Control NO PID AE Ver.vi"("Direction"=MOTOR_CONTROL_NO_PID_AE_DIRECTIONS_type_def."Stop", "AE Mode"=MOTOR_CONTROL_NO_PID_AE_DATA_ENTRY_MODE_Type_def."Write to motors") -> ()  [unwired: 3 in, 2 out]
      }
      frame "----SENSOR READING---- " {
      }
      frame "READ ENCODERS" {
        # ">>> Time cluster >>>"
        # ">>> Yaw >>>"
        # ">>> Stepper position >>>"
        # ">>> Object detection >>>"
        # ">>> Current encoder distance >>>"
        # ">>> Ultrasonic Sensors Detect >>>"
        n75 = call "Motor Control NO PID AE Ver.vi"("AE Mode"=MOTOR_CONTROL_NO_PID_AE_DATA_ENTRY_MODE_Type_def."Read from Encoders") -> ("Speed & distance"=w1260:T3)  [unwired: 4 in, 1 out]
        n76 = Unbundle By Name(w1260) -> ("xDistance"=w1259:dbl, "yDistance"=w1258:dbl, "wDistance"=w1257:dbl)
        n77 = Bundle By Name(cluster=w1265, "xDistance"=w1259, "yDistance"=w1258, "wDistance"=w1257) -> (w1264:T15)
      }
      frame "READ ULTRASONIC" {
        (unwired) navX_type_def."Read Values" ("Mode")
        (unwired) MOTOR_CONTROL_NO_PID_Type_Def."Latch" ("Direction")
        # ">>> Ultrasonic Sensors Detect >>>"
        # ">>> Object detection >>>"
        # ">>> Encoders >>>"
        # ">>> Stepper position >>>"
        # ">>> Yaw >>>"
        n78 = call "Arduino Interfacing VI.vi"("AE Mode"=Arduino_Interfacing."Read From Arduino") -> ("Arduino Data"=w1274:T5)  [unwired: 3 in, 1 out]
        n79 = Unbundle By Name(w1274) -> ("PING A"=w1273:u8, "PING B"=w1272:u8, "PING C"=w1271:u8, "PING D"=w1270:u8)
        n80 = Bundle By Name(cluster=w1280, "PING_A"=w1273, "PING_B"=w1272, "PING_C"=w1271, "PING_D"=w1270) -> (w1281:T14)
      }
      frame "READ YAW" {
        # ">>> Time cluster >>>"
        # ">>> Yaw >>>"
        # ">>> Ultrasonic Sensors Detect >>>"
        # ">>> Object detection >>>"
        # ">>> Encoders >>>"
        # ">>> Stepper position >>>"
        n81 = call "navX reading VI.vi"("Mode"=navX_type_def."Read Values") -> ("NavX Readings"=w1283:T4)  [unwired: 2 in, 3 out]
        n82 = Unbundle By Name(w1283) -> ("Heading"=w1282:dbl)
        n83 = Unbundle By Name(w1283) -> ("Yaw"=w1286:dbl)
        n84 = Bundle By Name(cluster=w1288, "Yaw"=w1286, "Compass"=w1282) -> (w1287:T11)
      }
      frame "----SYSTEM MODES----" {
        (unwired) I2C_MASTER_Type_Def."Last State" ("Arduino Mode")
        # ">>> Object detection >>>"
        # ">>> Yaw >>>"
        # ">>> Ultrasonic Sensors Detect >>>"
        # ">>> Encoders >>>"
        # ">>> Stepper position >>>"
      }
      frame "INIT" {
        w1318 = u8 0
        w1319 = 0.0
        # ">>> Time cluster >>>"
        # ">>> Object detection >>>"
        # ">>> Yaw >>>"
        # ">>> Ultrasonic Sensors Detect >>>"
        # ">>> Encoders >>>"
        # ">>> Stepper position >>>"
        # ">>State Logic  >>"
        n85 = call "Arduino Interfacing VI.vi"("AE Mode"=Arduino_Interfacing."Initialize") -> ()  [unwired: 3 in, 2 out]
        n86 = call "FGV Stop.vi"("Init/Read/Write State"=States_for_Action_Engine."Initialize") -> ()  [unwired: 2 in, 2 out]
        n87 = call "Motor Control NO PID AE Ver.vi"("AE Mode"=MOTOR_CONTROL_NO_PID_AE_DATA_ENTRY_MODE_Type_def."Initialize") -> ()  [unwired: 4 in, 2 out]
        n88 = call "Elasped Timer.vi"("Action"=Control."Initialize") -> ()  [unwired: 7 in, 4 out]
        n89 = Bundle By Name(cluster=w1312, "Recognized Object"=FALSE, "Object X coordinate"=0.0, "Object Y coordinate"=0.0) -> (w1311:T1)
        n90 = Bundle By Name(cluster=w1317, "y Stepper Position"=u8 0, "z Stepper Position"=u8 0) -> (w1316:T12)
        n91 = Bundle By Name(cluster=w1321, "xDistance"=w1319, "yDistance"=w1319, "wDistance"=w1319) -> (w1320:T15)
        n92 = Bundle By Name(cluster=w1323, "PING_A"=w1318, "PING_B"=w1318, "PING_C"=w1318, "PING_D"=w1318) -> (w1324:T14)
        n93 = Bundle By Name(cluster=w1307, "Yaw"=0.0) -> (w1306:T11)
      }
      frame "ARDUINO - ULTRASONIC" {
        # ">>> Object detection >>>"
        # ">>> Yaw >>>"
        # ">>> Ultrasonic Sensors Detect >>>"
        # ">>> Encoders >>>"
        # ">>> Stepper position >>>"
        # ">>State Logic  >>"
        n94 = call "Arduino Interfacing VI.vi"("Data to Write"=I2C_MASTER_WRITE_NEW_Type_Def."Ultrasonic sensors", "AE Mode"=Arduino_Interfacing."Write to Arduino") -> ()  [unwired: 2 in, 2 out]
      }
      frame "NAVX CALIBRATE" {
        # ">>> Object detection >>>"
        # ">>> Yaw >>>"
        # ">>> Ultrasonic Sensors Detect >>>"
        # ">>> Encoders >>>"
        # ">>> Stepper position >>>"
        # ">>State Logic  >>"
        # "Adds a 15 second delay to the startup process \nfor the NavX to calibrate"
        n95 = Wait (ms)(milliseconds to wait=u32 5000) -> ()  [unwired: 1 out]
      }
      frame "NO ACTION", Default {
        (unwired) u8 0 ("y Stepper value")
        (unwired) TRUE ("Latch")
        (unwired) navX_type_def."Read Values" ("Mode")
        (unwired) MOTOR_CONTROL_NO_PID_Type_Def."Latch" ("Direction")
        # ">>> Object detection >>>"
        # ">>> Yaw >>>"
        # ">>> Ultrasonic Sensors Detect >>>"
        # ">>> Encoders >>>"
        # ">>> Stepper position >>>"
        # ">>State Logic  >>"
        n96 = case shown="4" w1348 {
          tunnel: [0 100] -> w1350
          frame 1, Default {
          }
          frame 4 {
          }
        }
      }
      frame "----RESET CASES----" {
        (unwired) I2C_MASTER_Type_Def."Last State" ("Arduino Mode")
        # ">>> Object detection >>>"
        # ">>> Yaw >>>"
        # ">>> Ultrasonic Sensors Detect >>>"
        # ">>> Encoders >>>"
        # ">>> Stepper position >>>"
        # ">>State Logic  >>"
      }
      frame "RESET ENCODERS" {
        # ">>> Object detection >>>"
        # ">>> Yaw >>>"
        # ">>> Ultrasonic Sensors Detect >>>"
        # ">>> Encoders >>>"
        # ">>> Stepper position >>>"
        # ">>State Logic  >>"
        n97 = call "Motor Control NO PID AE Ver.vi"("AE Mode"=MOTOR_CONTROL_NO_PID_AE_DATA_ENTRY_MODE_Type_def."Reset Encoders") -> ()  [unwired: 4 in, 2 out]
      }
      frame "RESET FLAGS" {
        (unwired) I2C_MASTER_Type_Def."Last State" ("Arduino Mode")
        # "Resets any software variables\nand/or non-critical states"
        n98 = Wait (ms)(milliseconds to wait=u32 20) -> ()  [unwired: 1 out]
        n99 = Bundle By Name(cluster=w1372, "Time up flag"=FALSE, "SET TIME TO CHECK"=0.0) -> (w1371:T10)
        n100 = Bundle By Name(cluster=w1389, "Recognized Object"=FALSE, "Object X coordinate"=0.0, "Object Y coordinate"=0.0) -> (w1388:T1)
        n101 = Bundle By Name(cluster=w1379, "y Stepper Position"=u8 0, "z Stepper Position"=u8 0) -> (w1378:T12)
        n102 = Bundle By Name(cluster=w1384, "xDistance"=0.0, "yDistance"=0.0, "wDistance"=0.0) -> (w1383:T15)
        n103 = Bundle By Name(cluster=w1396, "PING_A"=u8 0, "PING_B"=u8 0, "PING_C"=u8 0, "PING_D"=u8 0) -> (w1395:T14)
        n104 = Bundle By Name(cluster=w1375, "Yaw"=0.0) -> (w1374:T11)
      }
      frame "RESET YAW" {
        n105 = Wait (ms)(milliseconds to wait=u32 100) -> ()  [unwired: 1 out]
        n106 = call "navX reading VI.vi"("Mode"=navX_type_def."Zero Yaw") -> ()  [unwired: 2 in, 4 out]
      }
      frame "RESET ARM" {
        n107 = call "Arduino Interfacing VI.vi"("Data to Write"=I2C_MASTER_WRITE_NEW_Type_Def."Soft Reset", "AE Mode"=Arduino_Interfacing."Write to Arduino") -> ()  [unwired: 2 in, 2 out]
      }
      frame "--------CAM STATES-------" {
      }
      frame "OPEN LOG CAM" {
        n108 = call "Webcam AE.vi"("Session In"=T29 "cam0", "Camera states"=Webcam_AE."Initialize Camera") -> ("error out"=w1425:errorcluster, "Session Out"=w1424:T29)  [unwired: 1 in, 1 out]
        n109 = call "Webcam AE.vi"("error in (no error)"=w1425, "Session In"=w1424, "Camera states"=Webcam_AE."Open Camera") -> ()  [unwired: 3 out]
      }
      frame "OPEN LIFE CAM" {
        n110 = call "Webcam AE.vi"("Session In"=T29 "cam1", "Camera states"=Webcam_AE."Initialize Camera") -> ("error out"=w1437:errorcluster, "Session Out"=w1436:T29)  [unwired: 1 in, 1 out]
        n111 = call "Webcam AE.vi"("error in (no error)"=w1437, "Session In"=w1436, "Camera states"=Webcam_AE."Open Camera") -> ()  [unwired: 3 out]
      }
      frame "CAM ACQ" {
        # ">>State Logic  >>"
        # ">>> Time cluster >>>"
        # ">>> Yaw >>>"
        # ">>> Stepper position >>>"
        # ">>> Encoders >>>"
        # ">>> Object detection >>>"
        # ">>> Ultrasonic Sensors Detect >>>"
        n112 = call "Webcam AE.vi"("error in (no error)"=w1447, "Camera states"=Webcam_AE."Continuous Acquisition") -> ()  [unwired: 1 in, 3 out]
      }
      frame "CAM CLOSE" {
        # ">>State Logic  >>"
        # ">>> Time cluster >>>"
        # ">>> Yaw >>>"
        # ">>> Stepper position >>>"
        # ">>> Encoders >>>"
        # ">>> Object detection >>>"
        # ">>> Ultrasonic Sensors Detect >>>"
        n113 = call "Webcam AE.vi"("Camera states"=Webcam_AE."Close Camera") -> ()  [unwired: 2 in, 3 out]
      }
      frame "PROCESS IMAGE" {
        # ">>State Logic  >>"
        # ">>> Time cluster >>>"
        # ">>> Yaw >>>"
        # ">>> Stepper position >>>"
        # ">>> Encoders >>>"
        # ">>> Object detection >>>"
        # ">>> Ultrasonic Sensors Detect >>>"
        n114 = call "Webcam AE.vi"("error in (no error)"=w1475, "Camera states"=Webcam_AE."Retrieve Image") -> ("error out"=w1471:errorcluster, "Image Out"=w1474:T23)  [unwired: 1 in, 1 out]
        n115 = call "Object Detection SubVI.vi"("Error In"=w1471, "Mode"="Object recognition mode", "Image Dest"=w1473, "Image in"=w1474) -> ("Object Center Coordinates"=w1468:cluster{"x":sgl, "y":sgl}, "Object detection cluster"=w1464:T2)  [unwired: 2 out]
        "Object detection cluster" <- w1464
        "Object Center Coordinates" <- w1468
        n116 = Unbundle By Name(w1464) -> ("Object detected?"=w1465:bool)
        n117 = Unbundle By Name(w1468) -> ("x"=w1467:sgl, "y"=w1466:sgl)
        n118 = Bundle By Name(cluster=w1470, "Recognized Object"=w1465, "Object X coordinate"=w1467, "Object Y coordinate"=w1466) -> (w1469:T1)
      }
      frame "DISPOSE BUFFERS" {
        # ">>State Logic  >>"
        # ">>> Time cluster >>>"
        # ">>> Yaw >>>"
        # ">>> Stepper position >>>"
        # ">>> Encoders >>>"
        # ">>> Object detection >>>"
        # ">>> Ultrasonic Sensors Detect >>>"
        n119 = call "Webcam AE.vi"("error in (no error)"=w1484, "Camera states"=Webcam_AE."Dispose Image Buffers") -> ()  [unwired: 1 in, 3 out]
      }
      frame "-----ARM ACTIONS-----" {
      }
      frame "CLOSE CLAW" {
        n120 = call "Arduino Interfacing VI.vi"("Data to Write"=I2C_MASTER_WRITE_NEW_Type_Def."Close Claw", "AE Mode"=Arduino_Interfacing."Write to Arduino") -> ()  [unwired: 2 in, 2 out]
      }
      frame "OPEN CLAW" {
        n121 = call "Arduino Interfacing VI.vi"("Data to Write"=I2C_MASTER_WRITE_NEW_Type_Def."Open Claw", "AE Mode"=Arduino_Interfacing."Write to Arduino") -> ()  [unwired: 2 in, 2 out]
      }
      frame "Z STEPPER CAM HEIGHT" {
        n122 = call "Arduino Interfacing VI.vi"("Data to Write"=I2C_MASTER_WRITE_NEW_Type_Def."zStepper 8k", "AE Mode"=Arduino_Interfacing."Write to Arduino") -> ()  [unwired: 2 in, 2 out]
      }
      frame "Z STEPPER GRAB HEIGHT" {
        # ">>State Logic  >>"
        # ">>> Time cluster >>>"
        # ">>> Yaw >>>"
        # ">>> Stepper position >>>"
        # ">>> Encoders >>>"
        # ">>> Object detection >>>"
        # ">>> Ultrasonic Sensors Detect >>>"
        n123 = call "Arduino Interfacing VI.vi"("Data to Write"=I2C_MASTER_WRITE_NEW_Type_Def."zStepper 100", "AE Mode"=Arduino_Interfacing."Write to Arduino") -> ()  [unwired: 2 in, 2 out]
      }
      frame "Y STEPPER CONTROL" {
        # ">>State Logic  >>"
        # ">>> yStepper command>>>"
        # ">>> Time cluster >>>"
        # ">>> Yaw >>>"
        # ">>> Stepper position >>>"
        # ">>> Encoders >>>"
        # ">>> Object detection >>>"
        # ">>> Ultrasonic Sensors Detect >>>"
        n124 = Unbundle By Name(w1536) -> ("yStepper desired"=w1535:u8)
        n125 = call "Arduino Interfacing VI.vi"("y Stepper value"=w1535, "Data to Write"=I2C_MASTER_WRITE_NEW_Type_Def."yStepper control", "AE Mode"=Arduino_Interfacing."Write to Arduino") -> ()  [unwired: 1 in, 2 out]
      }
      frame "READ STEPPER VALUES" {
        # ">>State Logic  >>"
        # ">>> Time cluster >>>"
        # ">>> Yaw >>>"
        # ">>> Stepper position >>>"
        # ">>> Encoders >>>"
        # ">>> Object detection >>>"
        # ">>> Ultrasonic Sensors Detect >>>"
        n126 = call "Arduino Interfacing VI.vi"("AE Mode"=Arduino_Interfacing."Read From Arduino") -> ("Arduino Data"=w1550:T5)  [unwired: 3 in, 1 out]
        n127 = Unbundle By Name(w1550) -> ("y Stepper Position"=w1549:u8, "z Stepper Position"=w1548:u8)
        n128 = Bundle By Name(cluster=w1553, "y Stepper Position"=w1549, "z Stepper Position"=w1548) -> (w1552:T12)
      }
      frame " -----TIMING-----" {
        # ">>State Logic  >>"
        # ">>> Time cluster >>>"
        # ">>> Yaw >>>"
        # ">>> Stepper position >>>"
        # ">>> Encoders >>>"
        # ">>> Object detection >>>"
        # ">>> Ultrasonic Sensors Detect >>>"
      }
      frame "SET TIMER" {
        # ">>State Logic  >>"
        # ">>> Time cluster >>>"
        # ">>> Yaw >>>"
        # ">>> Stepper position >>>"
        # ">>> Encoders >>>"
        # ">>> Object detection >>>"
        # ">>> Ultrasonic Sensors Detect >>>"
        n129 = call "Elasped Timer.vi"("Time Setting"=5.0, "Action"=Control."Initialize") -> ()  [unwired: 6 in, 4 out]
        n130 = Bundle By Name(cluster=w1568, "Time up flag"=FALSE) -> (w1566:T10)
      }
      frame "START TIMER" {
        # ">>State Logic  >>"
        # ">>> Time cluster >>>"
        # ">>> Yaw >>>"
        # ">>> Stepper position >>>"
        # ">>> Encoders >>>"
        # ">>> Object detection >>>"
        # ">>> Ultrasonic Sensors Detect >>>"
        n131 = call "Elasped Timer.vi"("Action"=Control."Start") -> ("Time Out?!"=w1576:bool)  [unwired: 7 in, 3 out]
        n132 = Bundle By Name(cluster=w1578, "Time up flag"=w1576) -> (w1577:T10)
      }
    }
    "State Logic" <- w221
    n133 = local read "TASK ENABLE"() -> (w215:bool)
    n134 = Not(x=w215) -> (.not. x?=w214:bool)
    n135 = case shown="True" w222 {
      tunnel: w226 -> [w249 w280]
      tunnel: w230 -> [w245 w282]
      tunnel: [w249 w280] -> w235
      tunnel: [w245 w283] -> w234
      tunnel: w231 -> [_ w278]
      tunnel: w233 -> [_ w279]
      tunnel: w228 -> [w248 w285]
      tunnel: [w248 w285] -> w227
      tunnel: "STOP TASK" -> [_ w268]
      tunnel: w221 -> [w247 w284]
      tunnel: [w247 w281] -> w220
      tunnel: w217 -> [w246 w274]
      tunnel: [w246 w274] -> w216
      tunnel: w214 -> [_ w269]
      tunnel: [w244 w266] -> w213
      tunnel: w212 -> [w244 w265]
      tunnel: w208 -> [w243 w262]
      tunnel: [w243 w262] -> w207
      tunnel: w205 -> [w242 w258]
      tunnel: [w242 w258] -> w204
      tunnel: w202 -> [w241 w256]
      tunnel: [w241 w256] -> w201
      tunnel: w199 -> [w240 w254]
      tunnel: [w240 w254] -> w198
      tunnel: w197 -> [w239 w253]
      tunnel: [w239 w252] -> w196
      tunnel: [_ w250] -> w195
      frame False {
        # ">>> yStepper command>>>"
        # ">>> Time cluster >>>"
        # ">>> Yaw >>>"
        # ">>> Stepper position >>>"
        # ">>> Encoders >>>"
        # ">>> Object detection >>>"
        # ">>> Ultrasonic Sensors Detect >>>"
        # ">>> Time cluster >>>"
        # ">>> Yaw >>>"
        # ">>> Stepper position >>>"
        # ">>> Encoders >>>"
        # ">>> Object detection >>>"
        # ">>> Ultrasonic Sensors Detect >>>"
      }
      frame True {
        # ">>State Logic Queue Reference >>"
        # ">>Timeout>>"
        # ">>> yStepper command>>>"
        # ">>> Time cluster >>>"
        # ">>> Object detection >>>"
        # ">>> Yaw >>>"
        # ">>> Ultrasonic Sensors Detect >>>"
        # ">>> Encoders >>>"
        # ">>> Stepper position >>>"
        # ">>State Logic  >>"
        # ">>True Stop Next State >>"
        # ">>Action Queue>>"
        # ">> Manual override >>"
        # ">>> Time cluster >>>"
        # ">>> Yaw >>>"
        # ">>> Stepper position >>>"
        # ">>> Encoders >>>"
        # ">>> Object detection >>>"
        # ">>> Ultrasonic Sensors Detect >>>"
        # ">>Action Queue>>"
        # ">>State Logic Queue Reference >>"
        n136 = Or(x=w268, y=w269) -> (x .or. y?=w267:bool)
        n137 = Unbundle By Name(w256) -> ("Yaw"=w257:dbl, "Compass"=w251:dbl)
        n138 = Unbundle By Name(w254) -> ("Time up flag"=w255:bool)
        "Time up flag" <- w255
        n139 = Unbundle By Name(w258) -> ("y Stepper Position"=w260:u8, "z Stepper Position"=w259:u8)
        n140 = Unbundle By Name(w274) -> ("xDistance"=w271:dbl, "yDistance"=w272:dbl, "wDistance"=w273:dbl)
        n141 = Unbundle By Name(w262) -> ("Recognized Object"=w261:bool, "Object X coordinate"=w264:dbl, "Object Y coordinate"=w263:dbl)
        n142 = Unbundle By Name(w285) -> ("PING_A"=w277:u8, "PING_B"=w276:u8, "PING_C"=w275:u8, "PING_D"=w270:u8)
        n143 = case shown="24" w284 {
          tunnel: [w288 w294 w306 w315 w375 w388 w425 w472 w514 w566 w612 w651 w710 w754 w793 w837 w876 w900 w952 w994 w1033 w1085 w1127] -> w283
          tunnel: w282 -> [w288 w297 w307 w318 w377 w389 w426 w473 w520 w559 w615 w658 w700 w757 w799 w834 w875 w905 w951 w998 w1041 w1080 w1118]
          tunnel: [State_Type_Definitions,_for_0.26g_versions_and_later_2."Idle" ("Enum") State_Type_Definitions,_for_0.26g_versions_and_later_2."Idle" ("Enum") w302 w317 State_Type_Definitions,_for_0.26g_versions_and_later_2."Shutdown" ("Enum") w390 w428 w471 w515 w565 w613 w653 w709 w755 w800 w836 w877 w899 w953 w995 w1034 w1086 w1119] -> w281
          tunnel: w280 -> [_ _ w305 w321 _ w395 w438 w480 w519 w563 w616 w657 w707 w752 w798 w842 w874 w904 w949 w993 w1040 w1083 w1126]
          tunnel: w279 -> [_ _ _ w320 _ w394 w437 w479 w518 w562 w609 w656 w706 w751 w797 w841 w873 w903 w948 w991 w1039 w1082 w1124]
          tunnel: w278 -> [_ _ w304 w316 _ w393 w436 w478 w517 w561 w608 w655 w708 w753 w796 w840 _ w902 w947 w992 w1038 w1081 w1125]
          tunnel: w267 -> [_ _ _ _ _ w387 w427 w475 w513 w564 w614 w659 w701 w758 w794 w838 _ w901 w950 w999 w1037 w1084 w1122]
          tunnel: w277 -> [_ _ _ _ _ _ _ _ _ _ _ _ _ _ _ _ _ _ _ _ _ _ _]
          tunnel: w276 -> [_ _ _ _ _ _ w434 _ _ w555 w597 w649 _ w747 _ _ _ _ _ _ _ _ _]
          tunnel: w275 -> [_ _ _ _ _ _ w433 _ _ w556 w598 w650 _ w748 _ _ _ _ _ _ _ _ _]
          tunnel: w273 -> [_ _ _ _ _ _ _ w477 _ _ _ _ _ _ _ _ _ _ _ _ _ _ _]
          tunnel: w272 -> [_ _ _ _ _ w386 _ _ _ _ _ w654 _ _ _ _ _ _ _ _ _ _ _]
          tunnel: w271 -> [_ _ _ _ _ _ _ _ _ _ w603 _ _ _ _ _ _ _ _ _ _ _ _]
          tunnel: w270 -> [_ _ _ _ _ _ _ _ _ _ _ _ _ _ _ _ _ _ _ _ _ _ _]
          tunnel: [State_Type_Definitions,_for_0.26g_versions_and_later_2."Idle" ("Enum") State_Type_Definitions,_for_0.26g_versions_and_later_2."Idle" ("Enum") State_Type_Definitions,_for_0.26g_versions_and_later_2."Idle" ("Enum") State_Type_Definitions,_for_0.26g_versions_and_later_2."Idle" ("Enum") State_Type_Definitions,_for_0.26g_versions_and_later_2."Shutdown" ("Enum") w383 w424 w468 w512 w558 w611 w652 w711 w756 w792 w835 w878 w898 w954 w997 w1035 w1087 w1120] -> w266
          tunnel: w265 -> [_ _ w302 _ _ _ _ _ _ _ _ _ _ _ _ _ _ _ _ _ _ _ _]
          tunnel: w261 -> [_ _ _ _ _ _ _ _ _ _ _ _ _ _ _ _ _ _ _ _ _ _ w1121]
          tunnel: w264 -> [_ _ _ _ _ _ _ _ _ _ _ _ _ _ _ w833 _ _ _ _ _ _ _]
          tunnel: w263 -> [_ _ _ _ _ _ _ _ _ _ _ _ _ _ _ _ w869 w906 _ _ _ _ _]
          tunnel: w260 -> [_ _ _ _ _ _ _ _ _ _ _ _ _ _ _ _ _ w907 _ _ _ _ _]
          tunnel: w259 -> [_ _ _ _ _ _ _ _ w510 _ _ _ w704 _ _ _ _ _ w946 _ w1032 w1079 _]
          tunnel: w257 -> [_ _ _ _ _ _ _ _ _ _ _ _ _ _ _ _ _ _ _ _ _ _ _]
          tunnel: w255 -> [_ _ _ _ _ _ _ _ _ _ _ _ _ _ w790 _ _ _ _ w990 _ _ _]
          tunnel: w253 -> [w286 w292 w301 w313 w373 w382 w423 w467 w511 w557 w607 w648 w699 w749 w791 w843 w867 w909 w945 w996 w1036 w1076 w1117]
          tunnel: [w286 w291 w301 w313 w373 w382 w423 w467 w511 w557 w607 w648 w699 w749 w791 w843 w867 w908 w945 w996 w1036 w1076 w1117] -> w252
          tunnel: w251 -> [_ _ _ _ _ _ _ _ _ _ _ _ _ _ _ _ _ _ _ _ _ _ _]
          tunnel: [_ _ _ TRUE _ _ _ _ _ _ _ _ _ _ _ _ _ _ _ _ _ _ _] -> w250
          frame 0 {
            # ">>> yStepper command>>>"
          }
          frame 1 {
            # ">>> yStepper command>>>"
            n144 = for {
              shift-right: [w300] -> w294
              shift-left: w297 -> [w299]
              tunnel: string[] ["INIT", "RESET ARM", "RESET FLAGS", "RESET YAW", "NAVX CALIBRATE"] -> [w298] mode=indexing
              n145 = Enqueue Element(queue=w299, element=w298) -> (queue out=w300:refnum<queue>)  [unwired: 2 in, 2 out]
            }
            n146 = Bundle By Name(cluster=w292, "yStepper desired"=u8 0) -> (w291:T9)
          }
          frame 3 {
            # ">>> yStepper command>>>"
            n147 = Flush Queue(queue=w305, error in (no error)=w304) -> ()  [unwired: 3 out]
            n148 = for {
              shift-right: [w311] -> w306
              shift-left: w307 -> [w310]
              tunnel: string[] ["STOP", "RESET ENCODERS", "RESET YAW", "RESET ARM", "DISPOSE BUFFERS", "CAM CLOSE", ""] -> [w309] mode=indexing
              n149 = Enqueue Element(queue=w310, element=w309) -> (queue out=w311:refnum<queue>)  [unwired: 2 in, 2 out]
            }
          }
          frame 4, Default {
            (unwired) TRUE ("Green LED")
            # ">>> yStepper command>>>"
            n150 = Dequeue Element(queue=w321, timeout in ms (-1)=w320, error in (no error)=w316) -> (element=w319:T8)  [unwired: 3 out]
            n151 = case shown="\"Start Task 5\"" w319 {
              tunnel: [w323 w330 w337 w344 w351 w358 w365 w367] -> w315
              tunnel: w318 -> [w324 w331 w338 w345 w352 w359 w365 w368]
              tunnel: [State_Type_Definitions."Task 1" ("Enum") State_Type_Definitions."Task 2" ("Enum") State_Type_Definitions,_for_0.26g_versions_and_later_2."Task 3" ("Enum") State_Type_Definitions,_for_0.26g_versions_and_later_2."Task 4_A" ("Enum") State_Type_Definitions."Task 5_A" ("Enum") State_Type_Definitions,_for_0.26g_versions_and_later_2."Task 6_A" ("Enum") State_Type_Definitions,_for_0.26g_versions_and_later_2."Idle" ("Enum") State_Type_Definitions,_for_0.26g_versions_and_later_2."Shutdown" ("Enum")] -> w317
              frame "Start Task 1" {
                n152 = for {
                  shift-right: [w328] -> w323
                  shift-left: w324 -> [w327]
                  tunnel: string[] ["RESET ENCODERS", "RESET YAW", "FORWARD", "READ ENCODERS"] -> [w326] mode=indexing
                  n153 = Enqueue Element(queue=w327, element=w326) -> (queue out=w328:refnum<queue>)  [unwired: 2 in, 2 out]
                }
              }
              frame "Start Task 2" {
                n154 = for {
                  shift-right: [w335] -> w330
                  shift-left: w331 -> [w334]
                  tunnel: string[] ["RESET ENCODERS", "RESET YAW", "READ ULTRASONIC", "ARDUINO - ULTRASONIC"] -> [w333] mode=indexing
                  n155 = Enqueue Element(queue=w334, element=w333) -> (queue out=w335:refnum<queue>)  [unwired: 2 in, 2 out]
                }
              }
              frame "Start Task 3" {
                n156 = for {
                  shift-right: [w342] -> w337
                  shift-left: w338 -> [w341]
                  tunnel: string[] ["RESET ENCODERS", "READ ENCODERS", "R-ACW"] -> [w340] mode=indexing
                  n157 = Enqueue Element(queue=w341, element=w340) -> (queue out=w342:refnum<queue>)  [unwired: 2 in, 2 out]
                }
              }
              frame "Start Task 4" {
                n158 = for {
                  shift-right: [w349] -> w344
                  shift-left: w345 -> [w348]
                  tunnel: string[] ["RESET YAW", "RESET ENCODERS", "RESET ARM", "RESET FLAGS", "", ""] -> [w347] mode=indexing
                  n159 = Enqueue Element(queue=w348, element=w347) -> (queue out=w349:refnum<queue>)  [unwired: 2 in, 2 out]
                }
              }
              frame "Start Task 5" {
                n160 = for {
                  shift-right: [w356] -> w351
                  shift-left: w352 -> [w355]
                  tunnel: string[] ["RESET YAW", "RESET ENCODERS", "RESET FLAGS", "RESET ARM", "", ""] -> [w354] mode=indexing
                  n161 = Enqueue Element(queue=w355, element=w354) -> (queue out=w356:refnum<queue>)  [unwired: 2 in, 2 out]
                }
              }
              frame "Start Task 6" {
                n162 = for {
                  shift-right: [w363] -> w358
                  shift-left: w359 -> [w362]
                  tunnel: string[] ["OPEN LOG CAM ", "", "", "", "", ""] -> [w361] mode=indexing
                  n163 = Enqueue Element(queue=w362, element=w361) -> (queue out=w363:refnum<queue>)  [unwired: 2 in, 2 out]
                }
              }
              frame "None", Default {
              }
              frame "Exit" {
                n164 = for {
                  shift-right: [w372] -> w367
                  shift-left: w368 -> [w371]
                  tunnel: string[] ["STOP", "RESET ENCODERS", "RESET YAW", "EXIT"] -> [w370] mode=indexing
                  n165 = Enqueue Element(queue=w371, element=w370) -> (queue out=w372:refnum<queue>)  [unwired: 2 in, 2 out]
                }
              }
            }
          }
          frame 5 {
            # ">>> yStepper command>>>"
            n166 = for {
              shift-right: [w381] -> w375
              shift-left: w377 -> [w380]
              tunnel: string[] ["INIT", "RESET ENCODERS", "RESET FLAGS", "EXIT"] -> [w379] mode=indexing
              n167 = Enqueue Element(queue=w380, element=w379) -> (queue out=w381:refnum<queue>)  [unwired: 2 in, 2 out]
            }
          }
          frame 6 {
            # ">>> yStepper command>>>"
            # "Use 250"
            n168 = Dequeue Element(queue=w395, timeout in ms (-1)=w394, error in (no error)=w393) -> (element=w392:T8)  [unwired: 3 out]
            n169 = Greater?(x=w386, y=250.0) -> (0:w384:bool)
            n170 = Or(x=w384, y=w387) -> (x .or. y?=w391:bool)
            n171 = case shown="\"Exit\"" w392 {
              tunnel: w391 -> [w398 _]
              tunnel: [w402 State_Type_Definitions,_for_0.26g_versions_and_later_2."True Stop" ("Enum")] -> w390
              tunnel: w389 -> [w399 w417]
              tunnel: [w397 w416] -> w388
              tunnel: [State_Type_Definitions,_for_0.26g_versions_and_later_2."Idle" ("Enum") State_Type_Definitions,_for_0.26g_versions_and_later_2."Shutdown" ("Enum")] -> w383
              frame "None", Default {
                n172 = case shown="True" w398 {
                  tunnel: w399 -> [w405 w411]
                  tunnel: [w404 w409] -> w397
                  frame False {
                    n173 = for {
                      shift-right: [w407] -> w404
                      shift-left: w405 -> [w408]
                      tunnel: string[] ["READ ENCODERS", "READ YAW", "FORWARD"] ("element") -> [w406] mode=indexing
                      n174 = Enqueue Element(queue=w408, element=w406) -> (queue out=w407:refnum<queue>)  [unwired: 2 in, 2 out]
                    }
                  }
                  frame True {
                    n175 = for {
                      shift-right: [w413] -> w409
                      shift-left: w411 -> [w414]
                      tunnel: string[] ["RESET YAW", "RESET ENCODERS", "STOP", ""] -> [w412] mode=indexing
                      n176 = Enqueue Element(queue=w414, element=w412) -> (queue out=w413:refnum<queue>)  [unwired: 2 in, 2 out]
                    }
                  }
                }
                n177 = Select(t=State_Type_Definitions,_for_0.26g_versions_and_later_2."True Stop" ("Enum"), s=w398, f=State_Type_Definitions."Task 1" ("Enum")) -> (s? t:f=w402:u16)
              }
              frame "Exit" {
                n178 = for {
                  shift-right: [w421] -> w416
                  shift-left: w417 -> [w422]
                  tunnel: string[] ["STOP", "RESET ENCODERS", "RESET YAW", ""] -> [w420] mode=indexing
                  n179 = Enqueue Element(queue=w422, element=w420) -> (queue out=w421:refnum<queue>)  [unwired: 2 in, 2 out]
                }
              }
            }
          }
          frame 7 {
            w432 = u8 10 ("y")
            # ">>> yStepper command>>>"
            # ">>Object detected>>"
            n180 = Dequeue Element(queue=w438, timeout in ms (-1)=w437, error in (no error)=w436) -> (element=w435:T8)  [unwired: 3 out]
            n181 = Less?(x=w434, y=w432) -> (x < y?=w431:bool)
            n182 = Less?(x=w433, y=w432) -> (x < y?=w430:bool)
            n183 = Or(x=w431, y=w430) -> (x .or. y?=w429:bool)
            "Obstacle detected" <- w429
            n184 = case shown="\"None\", Default" w435 {
              tunnel: w429 -> [w442 _]
              tunnel: [w444 State_Type_Definitions,_for_0.26g_versions_and_later_2."True Stop" ("Enum")] -> w428
              tunnel: w427 -> [w443 _]
              tunnel: w426 -> [w441 w461]
              tunnel: [w440 w462] -> w425
              tunnel: [State_Type_Definitions,_for_0.26g_versions_and_later_2."Idle" ("Enum") State_Type_Definitions,_for_0.26g_versions_and_later_2."Shutdown" ("Enum")] -> w424
              frame "None", Default {
                n185 = case shown="True" w442 {
                  tunnel: w441 -> [w448 w455]
                  tunnel: [w449 w454] -> w440
                  frame False {
                    n186 = for {
                      tunnel: string[] ["READ ULTRASONIC", "STOP"] ("element") -> [w450] mode=indexing
                      shift-right: [w452] -> w449
                      shift-left: w448 -> [w451]
                      n187 = Enqueue Element(queue=w451, element=w450) -> (queue out=w452:refnum<queue>)  [unwired: 2 in, 2 out]
                    }
                  }
                  frame True {
                    n188 = for {
                      shift-right: [w457] -> w454
                      shift-left: w455 -> [w458]
                      tunnel: string[] ["REVERSE", "READ ULTRASONIC", "READ YAW"] -> [w456] mode=indexing
                      n189 = Enqueue Element(queue=w458, element=w456) -> (queue out=w457:refnum<queue>)  [unwired: 2 in, 2 out]
                    }
                  }
                }
                n190 = Select(t=State_Type_Definitions,_for_0.26g_versions_and_later_2."True Stop" ("Enum"), s=w443, f=State_Type_Definitions."Task 2" ("Enum")) -> (s? t:f=w444:u16)
              }
              frame "Exit" {
                n191 = for {
                  shift-right: [w465] -> w462
                  shift-left: w461 -> [w466]
                  tunnel: string[] ["STOP", "RESET ENCODERS", "RESET YAW", "ARDUINO MODE 0"] -> [w464] mode=indexing
                  n192 = Enqueue Element(queue=w466, element=w464) -> (queue out=w465:refnum<queue>)  [unwired: 2 in, 2 out]
                }
              }
            }
          }
          frame 11 {
            # ">>> yStepper command>>>"
            n193 = Dequeue Element(queue=w480, timeout in ms (-1)=w479, error in (no error)=w478) -> (element=w469:T8)  [unwired: 3 out]
            n194 = Greater?(x=w477, y=100.0) -> (0:w474:bool)
            n195 = Or(x=w474, y=w475) -> (x .or. y?=w470:bool)
            n196 = case shown="\"Exit\"" w469 {
              tunnel: w470 -> [w483 _]
              tunnel: [w487 State_Type_Definitions,_for_0.26g_versions_and_later_2."True Stop" ("Enum")] -> w471
              tunnel: w473 -> [w484 w503]
              tunnel: [w482 w502] -> w472
              tunnel: [State_Type_Definitions,_for_0.26g_versions_and_later_2."Idle" ("Enum") State_Type_Definitions,_for_0.26g_versions_and_later_2."Shutdown" ("Enum")] -> w468
              frame "None", Default {
                n197 = case shown="False" w483 {
                  tunnel: w484 -> [w490 w496]
                  tunnel: [w489 w494] -> w482
                  frame False {
                    n198 = for {
                      shift-right: [w492] -> w489
                      shift-left: w490 -> [w493]
                      tunnel: string[] ["READ ENCODERS", "R-ACW"] ("element") -> [w491] mode=indexing
                      n199 = Enqueue Element(queue=w493, element=w491) -> (queue out=w492:refnum<queue>)  [unwired: 2 in, 2 out]
                    }
                  }
                  frame True {
                    n200 = for {
                      shift-right: [w498] -> w494
                      shift-left: w496 -> [w499]
                      tunnel: string[] ["RESET YAW", "RESET ENCODERS", "STOP", "ARDUINO MODE 0"] -> [w497] mode=indexing
                      n201 = Enqueue Element(queue=w499, element=w497) -> (queue out=w498:refnum<queue>)  [unwired: 2 in, 2 out]
                    }
                  }
                }
                n202 = Select(t=State_Type_Definitions,_for_0.26g_versions_and_later_2."True Stop" ("Enum"), s=w483, f=State_Type_Definitions,_for_0.26g_versions_and_later_2."Task 3" ("Enum")) -> (s? t:f=w487:T7)
              }
              frame "Exit" {
                n203 = for {
                  shift-right: [w506] -> w502
                  shift-left: w503 -> [w507]
                  tunnel: string[] ["STOP", "RESET ENCODERS", "RESET YAW", ""] -> [w505] mode=indexing
                  n204 = Enqueue Element(queue=w507, element=w505) -> (queue out=w506:refnum<queue>)  [unwired: 2 in, 2 out]
                }
              }
            }
          }
          frame 12 {
            # ">> Stepper height reeached >>"
            # ">>> yStepper command>>>"
            # ">> Manual override >>"
            n205 = Dequeue Element(queue=w519, timeout in ms (-1)=w518, error in (no error)=w517) -> (element=w516:T8)  [unwired: 3 out]
            n206 = Equal?(x=w510, y=u8 80) -> (x = y?=w508:bool)
            n207 = case shown="\"None\", Default" w516 {
              tunnel: [w531 State_Type_Definitions,_for_0.26g_versions_and_later_2."True Stop" ("Enum")] -> w515
              tunnel: [w529 w546] -> w514
              tunnel: w520 -> [w528 _]
              tunnel: w513 -> [w522 _]
              tunnel: [State_Type_Definitions,_for_0.26g_versions_and_later_2."Idle" ("Enum") State_Type_Definitions,_for_0.26g_versions_and_later_2."Shutdown" ("Enum")] -> w512
              tunnel: w508 -> [w521 _]
              frame "None", Default {
                # ">> WIill proceed to part ii if not manual override >>"
                # ">>If ENABLE or Trigger is set to true>>"
                n208 = Or(x=w521, y=w522) -> (x .or. y?=w523:bool)
                n209 = case shown="True" w521 {
                  tunnel: [w534 w540] -> w529
                  tunnel: w528 -> [w533 w539]
                  frame False {
                    n210 = for {
                      shift-right: [w536] -> w534
                      shift-left: w533 -> [w537]
                      tunnel: string[] ["Z STEPPER CAM HEIGHT", "READ STEPPER VALUES"] ("element") -> [w535] mode=indexing
                      n211 = Enqueue Element(queue=w537, element=w535) -> (queue out=w536:refnum<queue>)  [unwired: 2 in, 2 out]
                    }
                  }
                  frame True {
                    n212 = for {
                      shift-right: [w542] -> w540
                      shift-left: w539 -> [w543]
                      tunnel: string[] ["ARDUINO - ULTRASONIC", "READ ULTRASONIC", "FORWARD", "", "", ""] -> [w541] mode=indexing
                      n213 = Enqueue Element(queue=w543, element=w541) -> (queue out=w542:refnum<queue>)  [unwired: 2 in, 2 out]
                    }
                  }
                }
                n214 = Select(t=State_Type_Definitions,_for_0.26g_versions_and_later_2."True Stop" ("Enum"), s=w522, f=State_Type_Definitions,_for_0.26g_versions_and_later_2."Task 4_B" ("Enum")) -> (s? t:f=w525:T7)
                n215 = Select(t=w525, s=w523, f=State_Type_Definitions,_for_0.26g_versions_and_later_2."Task 4_A" ("Enum")) -> (s? t:f=w531:T7)
              }
              frame "Exit" {
                n216 = for {
                  shift-right: [w549] -> w546
                  shift-left: _ -> [w550]
                  tunnel: string[] ["STOP", "RESET ENCODERS", "RESET YAW", ""] -> [w548] mode=indexing
                  n217 = Enqueue Element(queue=w550, element=w548) -> (queue out=w549:refnum<queue>)  [unwired: 2 in, 2 out]
                }
              }
            }
          }
          frame 13 {
            w554 = u8 10
            # ">> Path blocked >>"
            # ">>> yStepper command>>>"
            # ">> Manual override >>"
            n218 = Dequeue Element(queue=w563, timeout in ms (-1)=w562, error in (no error)=w561) -> (element=w560:T8)  [unwired: 3 out]
            n219 = Less?(x=w556, y=w554) -> (x < y?=w551:bool)
            n220 = Less?(x=w555, y=w554) -> (x < y?=w552:bool)
            n221 = And(x=w552, y=w551) -> (x .and. y?=w553:bool)
            n222 = case shown="\"None\", Default" w560 {
              tunnel: [w577 State_Type_Definitions,_for_0.26g_versions_and_later_2."True Stop" ("Enum")] -> w565
              tunnel: [w575 w592] -> w566
              tunnel: w559 -> [w574 _]
              tunnel: w564 -> [w568 _]
              tunnel: [State_Type_Definitions,_for_0.26g_versions_and_later_2."Idle" ("Enum") State_Type_Definitions,_for_0.26g_versions_and_later_2."Shutdown" ("Enum")] -> w558
              tunnel: w553 -> [w567 _]
              frame "None", Default {
                # ">> Manual override forces program to true stop >>"
                # ">>If ENABLE or Trigger is set to true>>"
                n223 = Or(x=w567, y=w568) -> (x .or. y?=w573:bool)
                n224 = case shown="False" w567 {
                  tunnel: [w580 w585] -> w575
                  tunnel: w574 -> [w579 w584]
                  frame False {
                    n225 = for {
                      shift-right: [w582] -> w580
                      shift-left: w579 -> [w583]
                      tunnel: string[] ["FORWARD", "READ ULTRASONIC", "READ YAW"] ("element") -> [w581] mode=indexing
                      n226 = Enqueue Element(queue=w583, element=w581) -> (queue out=w582:refnum<queue>)  [unwired: 2 in, 2 out]
                    }
                  }
                  frame True {
                    n227 = for {
                      shift-right: [w588] -> w585
                      shift-left: w584 -> [w589]
                      tunnel: string[] ["STOP", "RESET YAW", "RESET ENCODERS", "RESET FLAGS"] -> [w587] mode=indexing
                      n228 = Enqueue Element(queue=w589, element=w587) -> (queue out=w588:refnum<queue>)  [unwired: 2 in, 2 out]
                    }
                  }
                }
                n229 = Select(t=State_Type_Definitions,_for_0.26g_versions_and_later_2."True Stop" ("Enum"), s=w568, f=State_Type_Definitions,_for_0.26g_versions_and_later_2."Task 4_C" ("Enum")) -> (s? t:f=w570:T7)
                n230 = Select(t=w570, s=w573, f=State_Type_Definitions,_for_0.26g_versions_and_later_2."Task 4_B" ("Enum")) -> (s? t:f=w577:T7)
              }
              frame "Exit" {
                n231 = for {
                  shift-right: [w595] -> w592
                  shift-left: _ -> [w596]
                  tunnel: string[] ["STOP", "RESET ENCODERS", "RESET YAW", ""] -> [w594] mode=indexing
                  n232 = Enqueue Element(queue=w596, element=w594) -> (queue out=w595:refnum<queue>)  [unwired: 2 in, 2 out]
                }
              }
            }
          }
          frame 14 {
            w606 = u8 20
            # ">> xDistance travelled>>"
            # ">> Path NOT blocked >>"
            # ">>> yStepper command>>>"
            # ">> Manual override >>"
            n233 = Dequeue Element(queue=w616, timeout in ms (-1)=w609, error in (no error)=w608) -> (element=w610:T8)  [unwired: 3 out]
            n234 = Greater?(x=w598, y=w606) -> (0:w604:bool)
            n235 = Greater?(x=w603, y=150.0) -> (0:w601:bool)
            n236 = Greater?(x=w597, y=w606) -> (0:w605:bool)
            n237 = And(x=w605, y=w604) -> (x .and. y?=w600:bool)
            n238 = And(x=w601, y=w600) -> (x .and. y?=w599:bool)
            n239 = case shown="\"None\", Default" w610 {
              tunnel: [w627 State_Type_Definitions,_for_0.26g_versions_and_later_2."True Stop" ("Enum")] -> w613
              tunnel: [w625 w643] -> w612
              tunnel: w615 -> [w624 w640]
              tunnel: w614 -> [w618 _]
              tunnel: [State_Type_Definitions,_for_0.26g_versions_and_later_2."Idle" ("t") State_Type_Definitions,_for_0.26g_versions_and_later_2."Shutdown" ("Enum")] -> w611
              tunnel: w599 -> [w617 _]
              frame "None", Default {
                # ">> Manual override forces program to true stop >>"
                # ">>If ENABLE or Trigger is set to true>>"
                n240 = Or(x=w617, y=w618) -> (x .or. y?=w623:bool)
                n241 = case shown="True" w617 {
                  tunnel: [w630 w635] -> w625
                  tunnel: w624 -> [w628 w634]
                  frame False {
                    n242 = for {
                      shift-right: [w632] -> w630
                      shift-left: w628 -> [w633]
                      tunnel: string[] ["RIGHT", "READ YAW", "READ ENCODERS", "READ ULTRASONIC"] ("element") -> [w631] mode=indexing
                      n243 = Enqueue Element(queue=w633, element=w631) -> (queue out=w632:refnum<queue>)  [unwired: 2 in, 2 out]
                    }
                  }
                  frame True {
                    n244 = for {
                      shift-right: [w638] -> w635
                      shift-left: w634 -> [w639]
                      tunnel: string[] ["STOP", "RESET YAW", "RESET ENCODERS", "ARDUINO - ULTRASONIC"] -> [w637] mode=indexing
                      n245 = Enqueue Element(queue=w639, element=w637) -> (queue out=w638:refnum<queue>)  [unwired: 2 in, 2 out]
                    }
                  }
                }
                n246 = Select(t=State_Type_Definitions,_for_0.26g_versions_and_later_2."True Stop" ("Enum"), s=w618, f=State_Type_Definitions,_for_0.26g_versions_and_later_2."Task 4_D" ("Enum")) -> (s? t:f=w619:T7)
                n247 = Select(t=w619, s=w623, f=State_Type_Definitions,_for_0.26g_versions_and_later_2."Task 4_C" ("Enum")) -> (s? t:f=w627:T7)
              }
              frame "Exit" {
                n248 = for {
                  shift-right: [w646] -> w643
                  shift-left: w640 -> [w647]
                  tunnel: string[] ["STOP", "RESET ENCODERS", "RESET YAW", ""] -> [w645] mode=indexing
                  n249 = Enqueue Element(queue=w647, element=w645) -> (queue out=w646:refnum<queue>)  [unwired: 2 in, 2 out]
                }
              }
            }
          }
          frame 15 {
            w666 = u8 20
            # ">> yDistance travelled>>"
            # ">> Path blocked >>"
            # ">>> yStepper command>>>"
            # ">> Manual override >>"
            n250 = Dequeue Element(queue=w657, timeout in ms (-1)=w656, error in (no error)=w655) -> (element=w667:T8)  [unwired: 3 out]
            n251 = Less?(x=w650, y=w666) -> (x < y?=w664:bool)
            n252 = Greater?(x=w654, y=200.0) -> (0:w662:bool)
            n253 = Less?(x=w649, y=w666) -> (x < y?=w665:bool)
            n254 = And(x=w665, y=w664) -> (x .and. y?=w661:bool)
            n255 = Or(x=w662, y=w661) -> (x .or. y?=w660:bool)
            n256 = case shown="\"None\", Default" w667 {
              tunnel: [w678 State_Type_Definitions,_for_0.26g_versions_and_later_2."True Stop" ("Enum")] -> w653
              tunnel: [w676 w694] -> w651
              tunnel: w658 -> [w675 w691]
              tunnel: w659 -> [w669 _]
              tunnel: [State_Type_Definitions,_for_0.26g_versions_and_later_2."Idle" ("t") State_Type_Definitions,_for_0.26g_versions_and_later_2."Shutdown" ("Enum")] -> w652
              tunnel: w660 -> [w668 _]
              frame "None", Default {
                # ">> Manual override forces program to true stop >>"
                # ">>If ENABLE or Trigger is set to true>>"
                n257 = Or(x=w668, y=w669) -> (x .or. y?=w674:bool)
                n258 = case shown="False" w668 {
                  tunnel: [w681 w686] -> w676
                  tunnel: w675 -> [w679 w685]
                  frame False {
                    n259 = for {
                      shift-right: [w683] -> w681
                      shift-left: w679 -> [w684]
                      tunnel: string[] ["FORWARD", "READ YAW", "READ ENCODERS", "READ ULTRASONIC"] ("element") -> [w682] mode=indexing
                      n260 = Enqueue Element(queue=w684, element=w682) -> (queue out=w683:refnum<queue>)  [unwired: 2 in, 2 out]
                    }
                  }
                  frame True {
                    n261 = for {
                      shift-right: [w689] -> w686
                      shift-left: w685 -> [w690]
                      tunnel: string[] ["STOP", "RESET YAW", "RESET ENCODERS", "RESET FLAGS"] -> [w688] mode=indexing
                      n262 = Enqueue Element(queue=w690, element=w688) -> (queue out=w689:refnum<queue>)  [unwired: 2 in, 2 out]
                    }
                  }
                }
                n263 = Select(t=State_Type_Definitions,_for_0.26g_versions_and_later_2."True Stop" ("Enum"), s=w669, f=State_Type_Definitions,_for_0.26g_versions_and_later_2."True Stop" ("Enum")) -> (s? t:f=w670:T7)
                n264 = Select(t=w670, s=w674, f=State_Type_Definitions,_for_0.26g_versions_and_later_2."Task 4_D" ("Enum")) -> (s? t:f=w678:T7)
              }
              frame "Exit" {
                n265 = for {
                  shift-right: [w697] -> w694
                  shift-left: w691 -> [w698]
                  tunnel: string[] ["STOP", "RESET ENCODERS", "RESET YAW", ""] -> [w696] mode=indexing
                  n266 = Enqueue Element(queue=w698, element=w696) -> (queue out=w697:refnum<queue>)  [unwired: 2 in, 2 out]
                }
              }
            }
          }
          frame 13 {
            # ">>> yStepper command>>>"
            # ">> Manual override >>"
            n267 = Dequeue Element(queue=w707, timeout in ms (-1)=w706, error in (no error)=w708) -> (element=w705:T8)  [unwired: 3 out]
            n268 = Equal?(x=w704, y=u8 80) -> (x = y?=w702:bool)
            n269 = case shown="\"None\", Default" w705 {
              tunnel: [w718 State_Type_Definitions,_for_0.26g_versions_and_later_2."True Stop" ("Enum")] -> w709
              tunnel: [w721 w738] -> w710
              tunnel: [State_Type_Definitions,_for_0.26g_versions_and_later_2."Idle" ("Enum") State_Type_Definitions,_for_0.26g_versions_and_later_2."Shutdown" ("Enum")] -> w711
              tunnel: w702 -> [w717 _]
              tunnel: w701 -> [w716 _]
              tunnel: w700 -> [w712 w735]
              frame "None", Default {
                # "Stays in Task 5_A until stepper reaches desired \nheight"
                # "T: Go back to idle, F: Continue with task\""
                # ">> Manual override >>"
                n270 = case shown="False" w717 {
                  tunnel: [w725 w731] -> w721
                  tunnel: w712 -> [w723 w729]
                  frame False {
                    n271 = for {
                      tunnel: string[] ["Z STEPPER CAM HEIGHT", "READ STEPPER VALUES"] ("element") -> [w726] mode=indexing
                      shift-right: [w728] -> w725
                      shift-left: w723 -> [w727]
                      n272 = Enqueue Element(queue=w727, element=w726) -> (queue out=w728:refnum<queue>)  [unwired: 2 in, 2 out]
                    }
                  }
                  frame True {
                    n273 = for {
                      shift-right: [w733] -> w731
                      shift-left: w729 -> [w734]
                      tunnel: string[] ["ARDUINO - ULTRASONIC", "READ ULTRASONIC", ""] -> [w732] mode=indexing
                      n274 = Enqueue Element(queue=w734, element=w732) -> (queue out=w733:refnum<queue>)  [unwired: 2 in, 2 out]
                    }
                  }
                }
                n275 = Or(x=w717, y=w716) -> (x .or. y?=w719:bool)
                n276 = Select(t=State_Type_Definitions,_for_0.26g_versions_and_later_2."True Stop" ("Enum"), s=w716, f=State_Type_Definitions."Task 5 _B" ("Enum")) -> (s? t:f=w713:u16)
                n277 = Select(t=w713, s=w719, f=State_Type_Definitions."Task 5_A" ("Enum")) -> (s? t:f=w718:u16)
              }
              frame "Exit" {
                n278 = for {
                  shift-right: [w741] -> w738
                  shift-left: w735 -> [w742]
                  tunnel: string[] ["STOP", "RESET ENCODERS", "RESET YAW", "ARDUINO MODE 0"] -> [w740] mode=indexing
                  n279 = Enqueue Element(queue=w742, element=w740) -> (queue out=w741:refnum<queue>)  [unwired: 2 in, 2 out]
                }
              }
            }
          }
          frame 14 {
            w746 = u8 15 ("y")
            # ">>> yStepper command>>>"
            n280 = Less?(x=w748, y=w746) -> (x < y?=w744:bool)
            n281 = Dequeue Element(queue=w752, timeout in ms (-1)=w751, error in (no error)=w753) -> (element=w750:T8)  [unwired: 3 out]
            n282 = Less?(x=w747, y=w746) -> (x < y?=w745:bool)
            n283 = And(x=w745, y=w744) -> (x .and. y?=w743:bool)
            n284 = case shown="\"None\", Default" w750 {
              tunnel: [w765 State_Type_Definitions,_for_0.26g_versions_and_later_2."True Stop" ("Enum")] -> w755
              tunnel: [w768 w785] -> w754
              tunnel: [State_Type_Definitions,_for_0.26g_versions_and_later_2."Idle" ("Enum") State_Type_Definitions,_for_0.26g_versions_and_later_2."Shutdown" ("Enum")] -> w756
              tunnel: w758 -> [w764 _]
              tunnel: w757 -> [w760 w782]
              tunnel: w743 -> [_ _]
              tunnel: w743 -> [w759 _]
              frame "None", Default {
                # "Stays in Task 5_B until it has stopped in front of box"
                # "T: Go back to idle, F: Continue with task\""
                # ">> Manual override >>"
                n285 = case shown="True" w759 {
                  tunnel: [w772 w778] -> w768
                  tunnel: w760 -> [w770 w776]
                  frame False {
                    n286 = for {
                      tunnel: string[] ["FORWARD", "READ ULTRASONIC", "READ YAW"] ("element") -> [w773] mode=indexing
                      shift-right: [w775] -> w772
                      shift-left: w770 -> [w774]
                      n287 = Enqueue Element(queue=w774, element=w773) -> (queue out=w775:refnum<queue>)  [unwired: 2 in, 2 out]
                    }
                  }
                  frame True {
                    n288 = for {
                      shift-right: [w780] -> w778
                      shift-left: w776 -> [w781]
                      tunnel: string[] ["STOP", "RESET YAW", "RESET ENCODERS", "OPEN LOG CAM", "SET TIMER"] -> [w779] mode=indexing
                      n289 = Enqueue Element(queue=w781, element=w779) -> (queue out=w780:refnum<queue>)  [unwired: 2 in, 2 out]
                    }
                  }
                }
                n290 = Or(x=w759, y=w764) -> (x .or. y?=w766:bool)
                n291 = Select(t=State_Type_Definitions,_for_0.26g_versions_and_later_2."True Stop" ("Enum"), s=w764, f=State_Type_Definitions."Task 5_C" ("Enum")) -> (s? t:f=w761:u16)
                n292 = Select(t=w761, s=w766, f=State_Type_Definitions."Task 5 _B" ("Enum")) -> (s? t:f=w765:u16)
              }
              frame "Exit" {
                n293 = for {
                  shift-right: [w788] -> w785
                  shift-left: w782 -> [w789]
                  tunnel: string[] ["STOP", "RESET ENCODERS", "RESET YAW", "ARDUINO MODE 0"] -> [w787] mode=indexing
                  n294 = Enqueue Element(queue=w789, element=w787) -> (queue out=w788:refnum<queue>)  [unwired: 2 in, 2 out]
                }
              }
            }
          }
          frame 15 {
            # ">>> yStepper command>>>"
            # ">> Manual override >>"
            n295 = Dequeue Element(queue=w798, timeout in ms (-1)=w797, error in (no error)=w796) -> (element=w795:T8)  [unwired: 3 out]
            n296 = case shown="\"None\", Default" w795 {
              tunnel: [w805 State_Type_Definitions,_for_0.26g_versions_and_later_2."True Stop" ("Enum")] -> w800
              tunnel: [w808 w825] -> w793
              tunnel: [State_Type_Definitions,_for_0.26g_versions_and_later_2."Idle" ("Enum") State_Type_Definitions,_for_0.26g_versions_and_later_2."Shutdown" ("Enum")] -> w792
              tunnel: w794 -> [w802 _]
              tunnel: w799 -> [w804 w822]
              tunnel: w790 -> [w801 _]
              frame "None", Default {
                # ">> Is object in range? >>"
                # "Determines if object is in range to pick up"
                # ">> Manual override >>"
                n297 = case shown="True" w801 {
                  tunnel: [w812 w818] -> w808
                  tunnel: w804 -> [w810 w816]
                  frame False {
                    n298 = for {
                      tunnel: string[] ["CAM ACQ", "START TIMER"] ("element") -> [w813] mode=indexing
                      shift-right: [w815] -> w812
                      shift-left: w810 -> [w814]
                      n299 = Enqueue Element(queue=w814, element=w813) -> (queue out=w815:refnum<queue>)  [unwired: 2 in, 2 out]
                    }
                  }
                  frame True {
                    n300 = for {
                      shift-right: [w820] -> w818
                      shift-left: w816 -> [w821]
                      tunnel: string[] ["CAM CLOSE", "PROCESS IMAGE"] -> [w819] mode=indexing
                      n301 = Enqueue Element(queue=w821, element=w819) -> (queue out=w820:refnum<queue>)  [unwired: 2 in, 2 out]
                    }
                  }
                }
                n302 = Or(x=w801, y=w802) -> (x .or. y?=w806:bool)
                n303 = Select(t=State_Type_Definitions."Task 5_D" ("Enum"), s=w806, f=State_Type_Definitions."Task 5_C" ("Enum")) -> (s? t:f=w805:T24)
              }
              frame "Exit" {
                n304 = for {
                  shift-right: [w828] -> w825
                  shift-left: w822 -> [w829]
                  tunnel: string[] ["STOP", "RESET ENCODERS", "RESET YAW", "ARDUINO MODE 0"] -> [w827] mode=indexing
                  n305 = Enqueue Element(queue=w829, element=w827) -> (queue out=w828:refnum<queue>)  [unwired: 2 in, 2 out]
                }
              }
            }
          }
          frame 16 {
            # ">>Action Queue>>"
            # ">>> yStepper command>>>"
            n306 = Dequeue Element(queue=w842, timeout in ms (-1)=w841, error in (no error)=w840) -> (element=w839:T8)  [unwired: 3 out]
            n307 = In Range and Coerce(upper limit=270.0, x=w833, lower limit=280.0) -> ()  [unwired: 2 out]
            n308 = case shown="\"None\", Default" w839 {
              tunnel: [w851 State_Type_Definitions,_for_0.26g_versions_and_later_2."True Stop" ("Enum")] -> w836
              tunnel: [w854 w862] -> w837
              tunnel: [State_Type_Definitions,_for_0.26g_versions_and_later_2."Idle" ("Enum") State_Type_Definitions,_for_0.26g_versions_and_later_2."Shutdown" ("Enum")] -> w835
              tunnel: w838 -> [w844 _]
              tunnel: w834 -> [w850 w859]
              tunnel: TRUE -> [w849 _]
              frame "None", Default {
                # ">> Manual override >>"
                # ">> Is object in range? >>"
                # "Determines if object is in range to pick up"
                # ">> Manual override >>"
                n309 = Or(x=w849, y=w844) -> (x .or. y?=w852:bool)
                n310 = Select(t=State_Type_Definitions,_for_0.26g_versions_and_later_2."True Stop" ("Enum"), s=w844, f=State_Type_Definitions."Task 5_F" ("Enum")) -> (s? t:f=w846:u16)
                n311 = for {
                  tunnel: string[] ["PROCESS IMAGE", ""] ("element") -> [w856] mode=indexing
                  shift-right: [w858] -> w854
                  shift-left: w850 -> [w857]
                  n312 = Enqueue Element(queue=w857, element=w856) -> (queue out=w858:refnum<queue>)  [unwired: 2 in, 2 out]
                }
                n313 = Select(t=w846, s=w852, f=State_Type_Definitions."Task 5_F" ("Enum")) -> (s? t:f=w851:u16)
              }
              frame "Exit" {
                n314 = for {
                  shift-right: [w865] -> w862
                  shift-left: w859 -> [w866]
                  tunnel: string[] ["STOP", "RESET ENCODERS", "RESET YAW", "ARDUINO MODE 0"] -> [w864] mode=indexing
                  n315 = Enqueue Element(queue=w866, element=w864) -> (queue out=w865:refnum<queue>)  [unwired: 2 in, 2 out]
                }
              }
            }
          }
          frame 21 {
            # ">>> yStepper command>>>"
            # ">>Object in range to pick up?>"
            n316 = Dequeue Element(queue=w874, timeout in ms (-1)=w873) -> (element=w872:T8)  [unwired: 1 in, 3 out]
            n317 = In Range and Coerce(upper limit=270.0, x=w869, lower limit=280.0) -> (In Range?=w868:bool)  [unwired: 1 out]
            "Is object in range to pick up?" <- w868
            n318 = case shown="\"None\", Default" w872 {
              tunnel: [w883 State_Type_Definitions,_for_0.26g_versions_and_later_2."True Stop" ("Enum")] -> w877
              tunnel: [w885 w893] -> w876
              tunnel: [State_Type_Definitions,_for_0.26g_versions_and_later_2."Idle" ("Enum") State_Type_Definitions,_for_0.26g_versions_and_later_2."Shutdown" ("Enum")] -> w878
              tunnel: w875 -> [w881 w890]
              tunnel: w868 -> [w879 _]
              frame "None", Default {
                # "Stays in Task 5_B until it has stopped in front of box"
                n319 = for {
                  shift-right: [w888] -> w885
                  shift-left: w881 -> [w889]
                  tunnel: string[] ["SET TIMER", "", "", "", ""] -> [w887] mode=indexing
                  n320 = Enqueue Element(queue=w889, element=w887) -> (queue out=w888:refnum<queue>)  [unwired: 2 in, 2 out]
                }
                n321 = Select(t=State_Type_Definitions."Task 5G" ("Enum"), s=w879, f=State_Type_Definitions."Task 5F_Error" ("Enum")) -> (s? t:f=w883:T24)
              }
              frame "Exit" {
                n322 = for {
                  shift-right: [w896] -> w893
                  shift-left: w890 -> [w897]
                  tunnel: string[] ["STOP", "RESET ENCODERS", "RESET YAW", "ARDUINO MODE 0"] -> [w895] mode=indexing
                  n323 = Enqueue Element(queue=w897, element=w895) -> (queue out=w896:refnum<queue>)  [unwired: 2 in, 2 out]
                }
              }
            }
          }
          frame 22 {
            # ">>> yStepper command>>>"
            # ">> Checks if yStepper has reached target>>"
            n324 = Dequeue Element(queue=w904, timeout in ms (-1)=w903, error in (no error)=w902) -> (element=w913:T8)  [unwired: 3 out]
            n325 = formula code="if (pos >= 160 && pos <= 180)\ny = 25;\nif (pos >= 181 &&pos <= 200) \ny = 20;\n\nelse if (pos >= 201 && pos <= 240)\ny = 15;\n\nelse if (pos >= 241 && pos <= 280)\ny = 10;\n\nelse if (pos >= 281 && pos <= 300)\ny = 5;\n\nelse if (pos > 300)\ny = 0;\n\nelse if (pos == 0 || pos < 100)\ny = 0;"("pos"=w906) -> ("y"=w912:dbl)
            n326 = To Unsigned Byte Integer(number=w912) -> (unsigned 8bit integer=w911:u8)
            n327 = Equal?(x=w907, y=w911) -> (x = y?=w910:bool)
            n328 = case shown="\"None\", Default" w913 {
              tunnel: [w920 State_Type_Definitions,_for_0.26g_versions_and_later_2."True Stop" ("Enum")] -> w899
              tunnel: [w923 w940] -> w900
              tunnel: [State_Type_Definitions,_for_0.26g_versions_and_later_2."Idle" ("Enum") State_Type_Definitions,_for_0.26g_versions_and_later_2."Shutdown" ("Enum")] -> w898
              tunnel: w901 -> [w919 _]
              tunnel: w905 -> [w915 w937]
              tunnel: w910 -> [w914 _]
              frame "None", Default {
                # ">> T: Breaks out of state loop; F: Stays in loop>>"
                # ">> Manual override >>"
                # ">> Checks if yStepper has reached target>>"
                # "Stays in Task 5_C until time is up and object is detected"
                # "T: Go back to idle, F: Continue with task\""
                # ">> Manual override >>"
                n329 = case shown="True" w914 {
                  tunnel: [w927 w933] -> w923
                  tunnel: w915 -> [w925 w931]
                  frame False {
                    n330 = for {
                      tunnel: string[] ["Y STEPPER CONTROL", "READ STEPPER VALUES", ""] ("element") -> [w928] mode=indexing
                      shift-right: [w930] -> w927
                      shift-left: w925 -> [w929]
                      n331 = Enqueue Element(queue=w929, element=w928) -> (queue out=w930:refnum<queue>)  [unwired: 2 in, 2 out]
                    }
                  }
                  frame True {
                    n332 = for {
                      shift-right: [w935] -> w933
                      shift-left: w931 -> [w936]
                      tunnel: string[] ["Z STEPPER GRAB HEIGHT", "READ STEPPER VALUES", "SET TIMER"] -> [w934] mode=indexing
                      n333 = Enqueue Element(queue=w936, element=w934) -> (queue out=w935:refnum<queue>)  [unwired: 2 in, 2 out]
                    }
                  }
                }
                n334 = Or(x=w914, y=w919) -> (x .or. y?=w921:bool)
                n335 = Select(t=State_Type_Definitions,_for_0.26g_versions_and_later_2."True Stop" ("Enum"), s=w919, f=State_Type_Definitions."Task 5G" ("Enum")) -> (s? t:f=w916:u16)
                n336 = Select(t=w916, s=w921, f=State_Type_Definitions."Task 5F_Error" ("Enum")) -> (s? t:f=w920:u16)
              }
              frame "Exit" {
                n337 = for {
                  shift-right: [w943] -> w940
                  shift-left: w937 -> [w944]
                  tunnel: string[] ["STOP", "RESET ENCODERS", "RESET YAW", "ARDUINO MODE 0"] -> [w942] mode=indexing
                  n338 = Enqueue Element(queue=w944, element=w942) -> (queue out=w943:refnum<queue>)  [unwired: 2 in, 2 out]
                }
              }
            }
            n339 = Bundle By Name(cluster=w909, "yStepper desired"=w911) -> (w908:T9)
          }
          frame 23 {
            # ">>> yStepper command>>>"
            # ">> Manual override >>"
            n340 = Dequeue Element(queue=w949, timeout in ms (-1)=w948, error in (no error)=w947) -> (element=w957:T8)  [unwired: 3 out]
            n341 = Equal?(x=w946, y=u8 1) -> (x = y?=w955:bool)
            n342 = case shown="\"None\", Default" w957 {
              tunnel: [w964 State_Type_Definitions,_for_0.26g_versions_and_later_2."True Stop" ("Enum")] -> w953
              tunnel: [w967 w985] -> w952
              tunnel: [State_Type_Definitions,_for_0.26g_versions_and_later_2."Idle" ("Enum") State_Type_Definitions,_for_0.26g_versions_and_later_2."Shutdown" ("Enum")] -> w954
              tunnel: w955 -> [w963 _]
              tunnel: w950 -> [w962 _]
              tunnel: w951 -> [w958 w982]
              frame "None", Default {
                # "Stays in Task 5G until stepper reaches desired \nheight"
                # "T: Go back to idle, F: Continue with task\""
                # ">> Manual override >>"
                n343 = case shown="False" w963 {
                  selector: w963 -> [_ w975]
                  tunnel: [w971 w978] -> w967
                  tunnel: w958 -> [w969 w976]
                  frame False {
                    n344 = for {
                      tunnel: string[] ["Z STEPPER CAM HEIGHT", "READ STEPPER VALUES"] ("element") -> [w972] mode=indexing
                      shift-right: [w974] -> w971
                      shift-left: w969 -> [w973]
                      n345 = Enqueue Element(queue=w973, element=w972) -> (queue out=w974:refnum<queue>)  [unwired: 2 in, 2 out]
                    }
                  }
                  frame True {
                    n346 = for {
                      shift-right: [w980] -> w978
                      shift-left: w976 -> [w981]
                      tunnel: string[] ["SET TIMER", "CLOSE CLAW", ""] -> [w979] mode=indexing
                      n347 = Enqueue Element(queue=w981, element=w979) -> (queue out=w980:refnum<queue>)  [unwired: 2 in, 2 out]
                    }
                    "Does this get triged" <- w975
                  }
                }
                n348 = Or(x=w963, y=w962) -> (x .or. y?=w965:bool)
                n349 = Select(t=State_Type_Definitions,_for_0.26g_versions_and_later_2."True Stop" ("Enum"), s=w962, f=State_Type_Definitions."Task 5H" ("Enum")) -> (s? t:f=w959:u16)
                n350 = Select(t=w959, s=w965, f=State_Type_Definitions."Task 5G" ("Enum")) -> (s? t:f=w964:u16)
              }
              frame "Exit" {
                n351 = for {
                  shift-right: [w988] -> w985
                  shift-left: w982 -> [w989]
                  tunnel: string[] ["STOP", "RESET ENCODERS", "RESET YAW", "ARDUINO MODE 0"] -> [w987] mode=indexing
                  n352 = Enqueue Element(queue=w989, element=w987) -> (queue out=w988:refnum<queue>)  [unwired: 2 in, 2 out]
                }
              }
            }
          }
          frame 24 {
            # ">>> yStepper command>>>"
            # ">> Manual override >>"
            n353 = Dequeue Element(queue=w993, timeout in ms (-1)=w991, error in (no error)=w992) -> (element=w1000:T8)  [unwired: 3 out]
            n354 = case shown="\"None\", Default" w1000 {
              tunnel: [w1007 State_Type_Definitions,_for_0.26g_versions_and_later_2."True Stop" ("Enum")] -> w995
              tunnel: [w1010 w1027] -> w994
              tunnel: [State_Type_Definitions,_for_0.26g_versions_and_later_2."Idle" ("Enum") State_Type_Definitions,_for_0.26g_versions_and_later_2."Shutdown" ("Enum")] -> w997
              tunnel: w990 -> [w1006 _]
              tunnel: w999 -> [w1005 _]
              tunnel: w998 -> [w1001 w1024]
              frame "None", Default {
                # "Stays in Task 5G until stepper reaches desired \nheight"
                # "T: Go back to idle, F: Continue with task\""
                # ">> Manual override >>"
                n355 = case shown="False" w1006 {
                  tunnel: [w1014 w1020] -> w1010
                  tunnel: w1001 -> [w1012 w1018]
                  frame False {
                    n356 = for {
                      tunnel: string[] ["START TIMER", "CLOSE CLAW", "", ""] ("element") -> [w1015] mode=indexing
                      shift-right: [w1017] -> w1014
                      shift-left: w1012 -> [w1016]
                      n357 = Enqueue Element(queue=w1016, element=w1015) -> (queue out=w1017:refnum<queue>)  [unwired: 2 in, 2 out]
                    }
                  }
                  frame True {
                    n358 = for {
                      shift-right: [w1022] -> w1020
                      shift-left: w1018 -> [w1023]
                      tunnel: string[] ["READ STEPPER VALUES", "", ""] -> [w1021] mode=indexing
                      n359 = Enqueue Element(queue=w1023, element=w1021) -> (queue out=w1022:refnum<queue>)  [unwired: 2 in, 2 out]
                    }
                  }
                }
                n360 = Or(x=w1006, y=w1005) -> (x .or. y?=w1008:bool)
                "Does it leave this state?" <- w1008
                n361 = Select(t=State_Type_Definitions,_for_0.26g_versions_and_later_2."True Stop" ("Enum"), s=w1005, f=State_Type_Definitions."Task 5I" ("Enum")) -> (s? t:f=w1002:u16)
                n362 = Select(t=w1002, s=w1008, f=State_Type_Definitions."Task 5H" ("Enum")) -> (s? t:f=w1007:u16)
              }
              frame "Exit" {
                n363 = for {
                  shift-right: [w1030] -> w1027
                  shift-left: w1024 -> [w1031]
                  tunnel: string[] ["STOP", "RESET ENCODERS", "RESET YAW", "ARDUINO MODE 0"] -> [w1029] mode=indexing
                  n364 = Enqueue Element(queue=w1031, element=w1029) -> (queue out=w1030:refnum<queue>)  [unwired: 2 in, 2 out]
                }
              }
            }
          }
          frame 25 {
            # ">>> yStepper command>>>"
            # ">> Manual override >>"
            n365 = Dequeue Element(queue=w1040, timeout in ms (-1)=w1039, error in (no error)=w1038) -> (element=w1044:T8)  [unwired: 3 out]
            n366 = Equal?(x=w1032, y=u8 80) -> (x = y?=w1042:bool)
            "Stepper position reached?" <- w1042
            n367 = case shown="\"None\", Default" w1044 {
              tunnel: [w1051 State_Type_Definitions,_for_0.26g_versions_and_later_2."True Stop" ("Enum")] -> w1034
              tunnel: [w1054 w1071] -> w1033
              tunnel: [State_Type_Definitions,_for_0.26g_versions_and_later_2."Idle" ("Enum") State_Type_Definitions,_for_0.26g_versions_and_later_2."Shutdown" ("Enum")] -> w1035
              tunnel: w1042 -> [w1050 _]
              tunnel: w1037 -> [w1049 _]
              tunnel: w1041 -> [w1045 w1068]
              frame "None", Default {
                # "Stays in Task 5G until stepper reaches desired \nheight"
                # "T: Go back to idle, F: Continue with task\""
                # ">> Manual override >>"
                n368 = case shown="True" w1050 {
                  tunnel: [w1058 w1064] -> w1054
                  tunnel: w1045 -> [w1056 w1062]
                  frame False {
                    n369 = for {
                      tunnel: string[] ["Z STEPPER CAM HEIGHT", "READ STEPPER VALUES"] ("element") -> [w1059] mode=indexing
                      shift-right: [w1061] -> w1058
                      shift-left: w1056 -> [w1060]
                      n370 = Enqueue Element(queue=w1060, element=w1059) -> (queue out=w1061:refnum<queue>)  [unwired: 2 in, 2 out]
                    }
                  }
                  frame True {
                    n371 = for {
                      shift-right: [w1066] -> w1064
                      shift-left: w1062 -> [w1067]
                      tunnel: string[] ["OPEN CLAW", "READ STEPPER VALUES", "RESET YAW"] -> [w1065] mode=indexing
                      n372 = Enqueue Element(queue=w1067, element=w1065) -> (queue out=w1066:refnum<queue>)  [unwired: 2 in, 2 out]
                    }
                  }
                }
                n373 = Or(x=w1050, y=w1049) -> (x .or. y?=w1052:bool)
                n374 = Select(t=State_Type_Definitions,_for_0.26g_versions_and_later_2."True Stop" ("Enum"), s=w1049, f=State_Type_Definitions,_for_0.26g_versions_and_later_2."True Stop" ("Enum")) -> (s? t:f=w1046:T7)
                n375 = Select(t=w1046, s=w1052, f=State_Type_Definitions."Task 5I" ("Enum")) -> (s? t:f=w1051:u16)
              }
              frame "Exit" {
                n376 = for {
                  shift-right: [w1074] -> w1071
                  shift-left: w1068 -> [w1075]
                  tunnel: string[] ["STOP", "RESET ENCODERS", "RESET YAW", "ARDUINO MODE 0"] -> [w1073] mode=indexing
                  n377 = Enqueue Element(queue=w1075, element=w1073) -> (queue out=w1074:refnum<queue>)  [unwired: 2 in, 2 out]
                }
              }
            }
          }
          frame 24 {
            # ">>> yStepper command>>>"
            n378 = Dequeue Element(queue=w1083, timeout in ms (-1)=w1082, error in (no error)=w1081) -> (element=w1088:T8)  [unwired: 3 out]
            n379 = Equal?(x=w1079, y=u8 80) -> (x = y?=w1078:bool)
            n380 = case shown="\"None\", Default" w1088 {
              tunnel: [w1095 State_Type_Definitions,_for_0.26g_versions_and_later_2."True Stop" ("Enum")] -> w1086
              tunnel: [w1094 w1112] -> w1085
              tunnel: [State_Type_Definitions,_for_0.26g_versions_and_later_2."Idle" ("Enum") State_Type_Definitions,_for_0.26g_versions_and_later_2."Shutdown" ("Enum")] -> w1087
              tunnel: w1084 -> [w1090 _]
              tunnel: w1080 -> [w1092 _]
              tunnel: w1078 -> [w1089 _]
              frame "None", Default {
                n381 = case shown="True" w1089 {
                  tunnel: [w1100 w1106] -> w1094
                  tunnel: w1092 -> [w1098 w1104]
                  frame False {
                    n382 = for {
                      tunnel: string[] ["Z STEPPER CAM HEIGHT", "READ STEPPER VALUES"] ("element") -> [w1101] mode=indexing
                      shift-right: [w1103] -> w1100
                      shift-left: w1098 -> [w1102]
                      n383 = Enqueue Element(queue=w1102, element=w1101) -> (queue out=w1103:refnum<queue>)  [unwired: 2 in, 2 out]
                    }
                  }
                  frame True {
                    n384 = for {
                      shift-right: [w1108] -> w1106
                      shift-left: w1104 -> [w1109]
                      tunnel: string[] ["CAM ACQ", "OPEN LOG CAM"] -> [w1107] mode=indexing
                      n385 = Enqueue Element(queue=w1109, element=w1107) -> (queue out=w1108:refnum<queue>)  [unwired: 2 in, 2 out]
                    }
                  }
                }
                n386 = Or(x=w1089, y=w1090) -> (x .or. y?=w1091:bool)
                n387 = Select(t=State_Type_Definitions,_for_0.26g_versions_and_later_2."Task 6_B" ("Enum"), s=w1091, f=State_Type_Definitions,_for_0.26g_versions_and_later_2."Task 6_A" ("Enum")) -> (s? t:f=w1095:T7)
              }
              frame "Exit" {
                n388 = for {
                  shift-right: [w1115] -> w1112
                  shift-left: _ -> [w1116]
                  tunnel: string[] ["STOP", "RESET ENCODERS", "RESET YAW", "ARDUINO MODE 0"] -> [w1114] mode=indexing
                  n389 = Enqueue Element(queue=w1116, element=w1114) -> (queue out=w1115:refnum<queue>)  [unwired: 2 in, 2 out]
                }
              }
            }
          }
          frame 25 {
            # ">>> yStepper command>>>"
            n390 = Dequeue Element(queue=w1126, timeout in ms (-1)=w1124, error in (no error)=w1125) -> (element=w1123:T8)  [unwired: 3 out]
            n391 = case shown="\"None\", Default" w1123 {
              tunnel: [w1133 State_Type_Definitions,_for_0.26g_versions_and_later_2."True Stop" ("Enum")] -> w1119
              tunnel: [w1132 w1151] -> w1127
              tunnel: [State_Type_Definitions,_for_0.26g_versions_and_later_2."Idle" ("Enum") State_Type_Definitions,_for_0.26g_versions_and_later_2."Shutdown" ("Enum")] -> w1120
              tunnel: w1122 -> [w1128 _]
              tunnel: w1121 -> [w1130 _]
              tunnel: w1118 -> [w1129 w1148]
              frame "None", Default {
                # ">> Manual override >>"
                n392 = case shown="True" w1130 {
                  tunnel: [w1138 w1144] -> w1132
                  tunnel: w1129 -> [w1137 w1142]
                  frame False {
                    n393 = for {
                      shift-right: [w1141] -> w1138
                      shift-left: w1137 -> [w1140]
                      tunnel: string[] ["CAM ACQ", "PROCESS IMAGE", "OPEN CLAW"] -> [w1139] mode=indexing
                      n394 = Enqueue Element(queue=w1140, element=w1139) -> (queue out=w1141:refnum<queue>)  [unwired: 2 in, 2 out]
                    }
                  }
                  frame True {
                    n395 = for {
                      shift-right: [w1146] -> w1144
                      shift-left: w1142 -> [w1147]
                      tunnel: string[] ["CAM ACQ", "PROCESS IMAGE", "CLOSE CLAW"] -> [w1145] mode=indexing
                      n396 = Enqueue Element(queue=w1147, element=w1145) -> (queue out=w1146:refnum<queue>)  [unwired: 2 in, 2 out]
                    }
                  }
                }
                n397 = Select(t=State_Type_Definitions,_for_0.26g_versions_and_later_2."True Stop" ("Enum"), s=w1128, f=State_Type_Definitions,_for_0.26g_versions_and_later_2."Task 6_B" ("Enum")) -> (s? t:f=w1133:T7)
              }
              frame "Exit" {
                # ">> State after true stop >>"
                # ">> Goes to true stop >>"
                n398 = for {
                  shift-right: [w1154] -> w1151
                  shift-left: w1148 -> [w1155]
                  tunnel: string[] ["STOP", "RESET ENCODERS", "RESET YAW", ""] -> [w1153] mode=indexing
                  n399 = Enqueue Element(queue=w1155, element=w1153) -> (queue out=w1154:refnum<queue>)  [unwired: 2 in, 2 out]
                }
              }
            }
          }
        }
        "Cluster" <- w262
      }
    }
    n400 = local write "Green LED"(w195) -> ()
  }
  n401 = call <vilib>:"DIO Close.vi"("error in (no error)"=w24, "DIO Info In"=w27) -> ()  [unwired: 9 in, 1 out]
  n402 = call <vilib>:"DIO Close.vi"("error in (no error)"=w34, "DIO Info In"=w36) -> ()  [unwired: 9 in, 1 out]
  n403 = call <vilib>:"NavX Close.vi"("error in (no error)"=w5, "NavX Info In"=w4) -> ()  [unwired: 9 in, 1 out]
  n404 = call <vilib>:"DIO Close.vi"("error in (no error)"=w29, "DIO Info In"=w31) -> ()  [unwired: 9 in, 1 out]
  n405 = call <vilib>:"DIO Close.vi"("error in (no error)"=w12, "DIO Info In"=w13) -> ()  [unwired: 9 in, 1 out]
  n406 = call <vilib>:"DIO Close.vi"("error in (no error)"=w7, "DIO Info In"=w8) -> ()  [unwired: 9 in, 1 out]
  n407 = while {
    stop <- w1587 stop-if-true
    n408 = call <vilib>:"RT Get CPU Loads.vi"() -> ("CPU loads"=→"CPU loads":T6[])  [unwired: 10 in, 1 out]
    n409 = Wait (ms)(milliseconds to wait=u32 100) -> ()  [unwired: 1 out]
    n410 = call "FGV Stop.vi"("Init/Read/Write State"=States_for_Action_Engine."Read") -> ("Output node"=w1587:bool)  [unwired: 2 in, 1 out]
  }
  n411 = Merge Errors "Merge Errors"(w63, w62) -> (w45:errorcluster)
  n412 = Merge Errors(w49, w45) -> (w44:errorcluster)
  n413 = Destroy User Event(user event=w66, error in=w44) -> ()  [unwired: 1 out]
  n414 = Destroy User Event(user event=w67, error in=w44) -> ()  [unwired: 1 out]
  n415 = Unregister For Events(event registration refnum=w58, error in=w44) -> ()  [unwired: 1 out]
  n416 = Release Queue(queue=w40, error in (no error)=w44) -> (error out=w23:errorcluster)  [unwired: 1 in, 2 out]
  n417 = Release Queue(queue=w57, error in (no error)=w44) -> ()  [unwired: 1 in, 3 out]
  n418 = call <vilib>:"Simple Error Handler.vi"("error in (no error)"=w23) -> ("error out"=w22:errorcluster)  [unwired: 4 in, 4 out]
  n419 = call <vilib>:"Reset myRIO.vi"("error in (no error)"=w22) -> ("error out"=→"error out":errorcluster)  [unwired: 10 in]
